vi "Main_MaintenanceCountersV1.vi"() -> ()   [LabVIEW 2017]
panel:
  out "HourResetEnabled":string
  out "CycleCountHour":T1
  in  "ArrayCycleCountHour":T2(array[cluster])
  out "UserLevel":i32
  out "ServerConnectionStatus":string
  out "Line Name":string
  out "Array_BooleanMemoryPLC":T3(array[cluster])
  out "UserLogged":string
  in  "FormatCountersConfigArray":T4(array[cluster]) {"StoppageAlarmCounter" format="%#_6f"; "PreparationAlarmCounter" format="%#_6f"}
  out "CycleTimeCluster":T5
  out "Table Control":string[][](table)
  out "ConnectionCluster":cluster{"Connection":bool, "MachineName":string}
  out "UDT_1":T6
  in  "CountersConfiguration":T7
  out "CountersConfigMerged":T4(array[cluster])
  out "CounterLineName Path":path
  in  "stop":bool
  in  "Tab":T8(tab)
  in  "RefreshLists":bool
  in  "Selector_P#-Description":u16(ring) items=["104567 - Spinning Belt", "108724 - Emergency Stop", "105855 - Helicoil", "101415 - Inductive Sensor", "101111 - Magnetic Sensor"]
  in  "Selector_MachineSpareParts":u16(ring) items=["MA530", "MA520", "MA500-3", "MA500-2", "MA500-1", "MA490-2", "MA490-1", "MA475", "MA470", "MA455", "MA336", "MA335"]
  out "PathLocationMachineImage":path
  out "PathSparePartImage":path
  out "Image_LocationInMachine":T9(plugin-control)
  out "Image_SparePart":T9(plugin-control)
  in  "CountersConfigArray":T4(array[cluster]) {"StoppageAlarmCounter" format="%#_6f"; "PreparationAlarmCounter" format="%#_6f"}
  in  "RefreshCountersConfig":bool
  in  "SaveCountersConfig":bool
  out "Counters Configuration Path":path
  in  "MachineNameID":u16(ring) items=["MA530", "MA520", "MA500-3", "MA500-2", "MA500-1", "MA490-2", "MA490-1", "MA475", "MA470", "MA455", "MA336", "MA335"]
  in  "PLC Connection Array":T10(array[cluster]) {"MemoryType 3" items=["CR (Control Relay)"=1, "MR (Internal Auxiliary Relay)"=2, "VB (Work Relay)"=3, "LR (Latch Relay)"=4, "B (Link Relay)"=5, "R (Relay)"=6, "DM (Data Memory)"=7, "EM (Extended Data Memory)"=8, "FM (File Register 1)"=9, "ZF (FIle Register 2)"=10, "W (Link Register)"=11, "TM (Temporary Data Memory)"=12, "Z (Index Register)"=13, "T (Timer)"=14, "TC (Timer (Counter Value))"=15, "TS (Timer Set Value)"=16, "C (Counter)"=17, "CC (Counter (Counter Value))"=18, "CS (Counter (Set Value))"=19, "CTH (High Speed Counter)"=20, "CTC (High Speed Counter Comparator (Set Value))"=21, "AT (Digital Trimmer)"=22, "CM (Control Memory)"=23, "VM (Work Memory)"=24]; "MemoryType 2" items=["CR (Control Relay)"=1, "MR (Internal Auxiliary Relay)"=2, "VB (Work Relay)"=3, "LR (Latch Relay)"=4, "B (Link Relay)"=5, "R (Relay)"=6, "DM (Data Memory)"=7, "EM (Extended Data Memory)"=8, "FM (File Register 1)"=9, "ZF (FIle Register 2)"=10, "W (Link Register)"=11, "TM (Temporary Data Memory)"=12, "Z (Index Register)"=13, "T (Timer)"=14, "TC (Timer (Counter Value))"=15, "TS (Timer Set Value)"=16, "C (Counter)"=17, "CC (Counter (Counter Value))"=18, "CS (Counter (Set Value))"=19, "CTH (High Speed Counter)"=20, "CTC (High Speed Counter Comparator (Set Value))"=21, "AT (Digital Trimmer)"=22, "CM (Control Memory)"=23, "VM (Work Memory)"=24]; "MemoryType" items=["CR (Control Relay)"=1, "MR (Internal Auxiliary Relay)"=2, "VB (Work Relay)"=3, "LR (Latch Relay)"=4, "B (Link Relay)"=5, "R (Relay)"=6, "DM (Data Memory)"=7, "EM (Extended Data Memory)"=8, "FM (File Register 1)"=9, "ZF (FIle Register 2)"=10, "W (Link Register)"=11, "TM (Temporary Data Memory)"=12, "Z (Index Register)"=13, "T (Timer)"=14, "TC (Timer (Counter Value))"=15, "TS (Timer Set Value)"=16, "C (Counter)"=17, "CC (Counter (Counter Value))"=18, "CS (Counter (Set Value))"=19, "CTH (High Speed Counter)"=20, "CTC (High Speed Counter Comparator (Set Value))"=21, "AT (Digital Trimmer)"=22, "CM (Control Memory)"=23, "VM (Work Memory)"=24]; "PLC Type" items=["Keyence", "Allen Bradley", "Mitsubishi", "Panasonic", "Siemens"]}
  out "PLC Configuration Path":path
  in  "SavePLCConfig":bool
  in  "RefreshPLCConfig":bool
  in  "CreateTables":bool
  in  "EditUser":bool
  in  "GeneralParametersArray":cluster{"Parameter":string, "Value":string}[](array[cluster])
  in  "LoadDefaultConfig":bool
  in  "RemoveUser":bool
  in  "Logout":bool
  in  "Login":bool
  in  "AddUser":bool
  in  "GDrive":bool
  out "GeneralConfigPath":path
  in  "RefreshGeneralConfig":bool
  in  "SaveGeneralConfig":bool
  in  "ShowParetto":bool
  out "CycleTimeMonitor":T11(array[cluster])
  out "CycleTimePath":path
  out "legend":string[][](table)
  in  "Tab Control":T12(tab)
  in  "DictionaryArray":T13(array[cluster]) {"LifeCycle" format="%#_6f"}
  out "PathDictionary":path
  in  "SaveDictionary":bool
  in  "RefreshDictionary":bool
  in  "ResetAlarmButton":bool
  in  "QualityLogin":bool
  in  "MaintenanceLogin":bool
  in  "ResetAlarm":bool[](array[boolean])
  out "ArrayAlarm":bool[](array[boolean])
  out "OnlineStations":T14(array[cluster])
  in  "Counters Monitor Array":T15(array[cluster])
  out "CurrentCountersPath":path
  in  "Count Signal":bool[](array[boolean])
  in  "SaveCurrentCounter":bool
  in  "RefreshCurrentCounter":bool
  in  "Sort":bool
  out "Hour":string
  # "Cycles Based Maintenance"
  # "1. Save counters to be loaded in the last state when the app starts up.\n\n2.Algorithm to read PLC counter values.\nthe key will be to set the signal from the PLC and reset from LabVIEW and the machine won't be able to start the new signal if the application has not been reset the previous one.\n\n3. Autosort getting the red status all the way up.\n\n4. Check cyle time between parts (The count signal must is the same for all the components in the same machine)"
  # "User"
  # "Line"
  # "Nidec Server Connection"
  # "buscar multiplos de ciclos para que coincidan \n\nestudiar investigacion de operaciones\n\nAgrupar las maquinas que trabajan en conjunto para agrupar tareas de mantenimiento.\nCambiar el metodo de seleccion de memorias de PLC usando solo strings para hacerlos universales."
  # "Nota para desarrollador: Revisar que al cerrar la incidencia se apague la alarma y se resetee el contador"
  # "Refresh Lists"
  # "Select Machine"
  # "Select PartNumber - Description"
  # "Spare Part Image"
  # "Location in the Machine"
  # "These paths are calculated automatically"
  # "Machine Name"
  # "Tool Crib P#"
  # "Description"
  # "SP1"
  # "SP2"
  # "Note:\nSP1 = Is the setpoint for the counter when the \nmachine will alert to prepare the replacement of\nthe component. This gives the technician time\nto get parts together.\n\nSP2 = Is the setpoint for the counter when the\nmachine will stop the operation until the part is \nreplaced, the operation can only be reset until\na quality employee comes to unlock with its \nuser and password."
  # "USER LEVEL 3 OR ABOVE TO ENABLE THIS CONFIGURATION IS NEEDED."
  # "Count Signal"
  # "Alarm Signal"
  # "Alarm Message"
  # "Add the option to connect by serial port"
  # "Machine Name"
  # "PLC Address"
  # "PLC Type"
  # "Memory Type"
  # "Number"
  # "Memory Type"
  # "Number"
  # "Number"
  # "Memory Type"
  # "Value"
  # "Parameter"
  # "User Level 5 Requiered to View General Parameters"
  # "User Management"
  # "Idle Time: Is the maximum waiting time before a breakdown incidence is\nconsidered and created."
  # "Escalation Time: Is the maximum waiting time before sending an email \nto the escalation chain."
  # "Cycle Time Monitor"
  # "Cycle Time Monitor"
  # "Note: \nTo add a machine in this list of counters configuration it must be firt added in the PLC Connection tab."
  # "The SubAssembly can be either EOL, Motor, Stator, Rotor Etc, This is used to be able to crate several tables for the same line."
  # "Component"
  # "Cycle Life"
  # "Manual"
  # "Un calculador de tiempo de vida en ciclos, que dependa del tipo de componente para calcular de acuerdo a la aplicacion.\n\npor ejemplo un slider, su tiempo de vida en es km de recorrido, midiendo cuanto se desplaza en cada movimiento, y cuantos desplazamientos hace por ciclo, se puede predecir, a los cuantos\nciclos va a fallar."
  # "Version:\nCBM V1.0\n02/19/2022\nEdgar Cruz\nMaintenance"
  # "Online Stations"
  # "MachineName"
  # "Tool Crib"
  # "ComponentName"
  # "Counter SetPoint"
  # "Actual"
  # "Status"
  # "Maintenance"
  # "Quality"
  # "Current Hour"
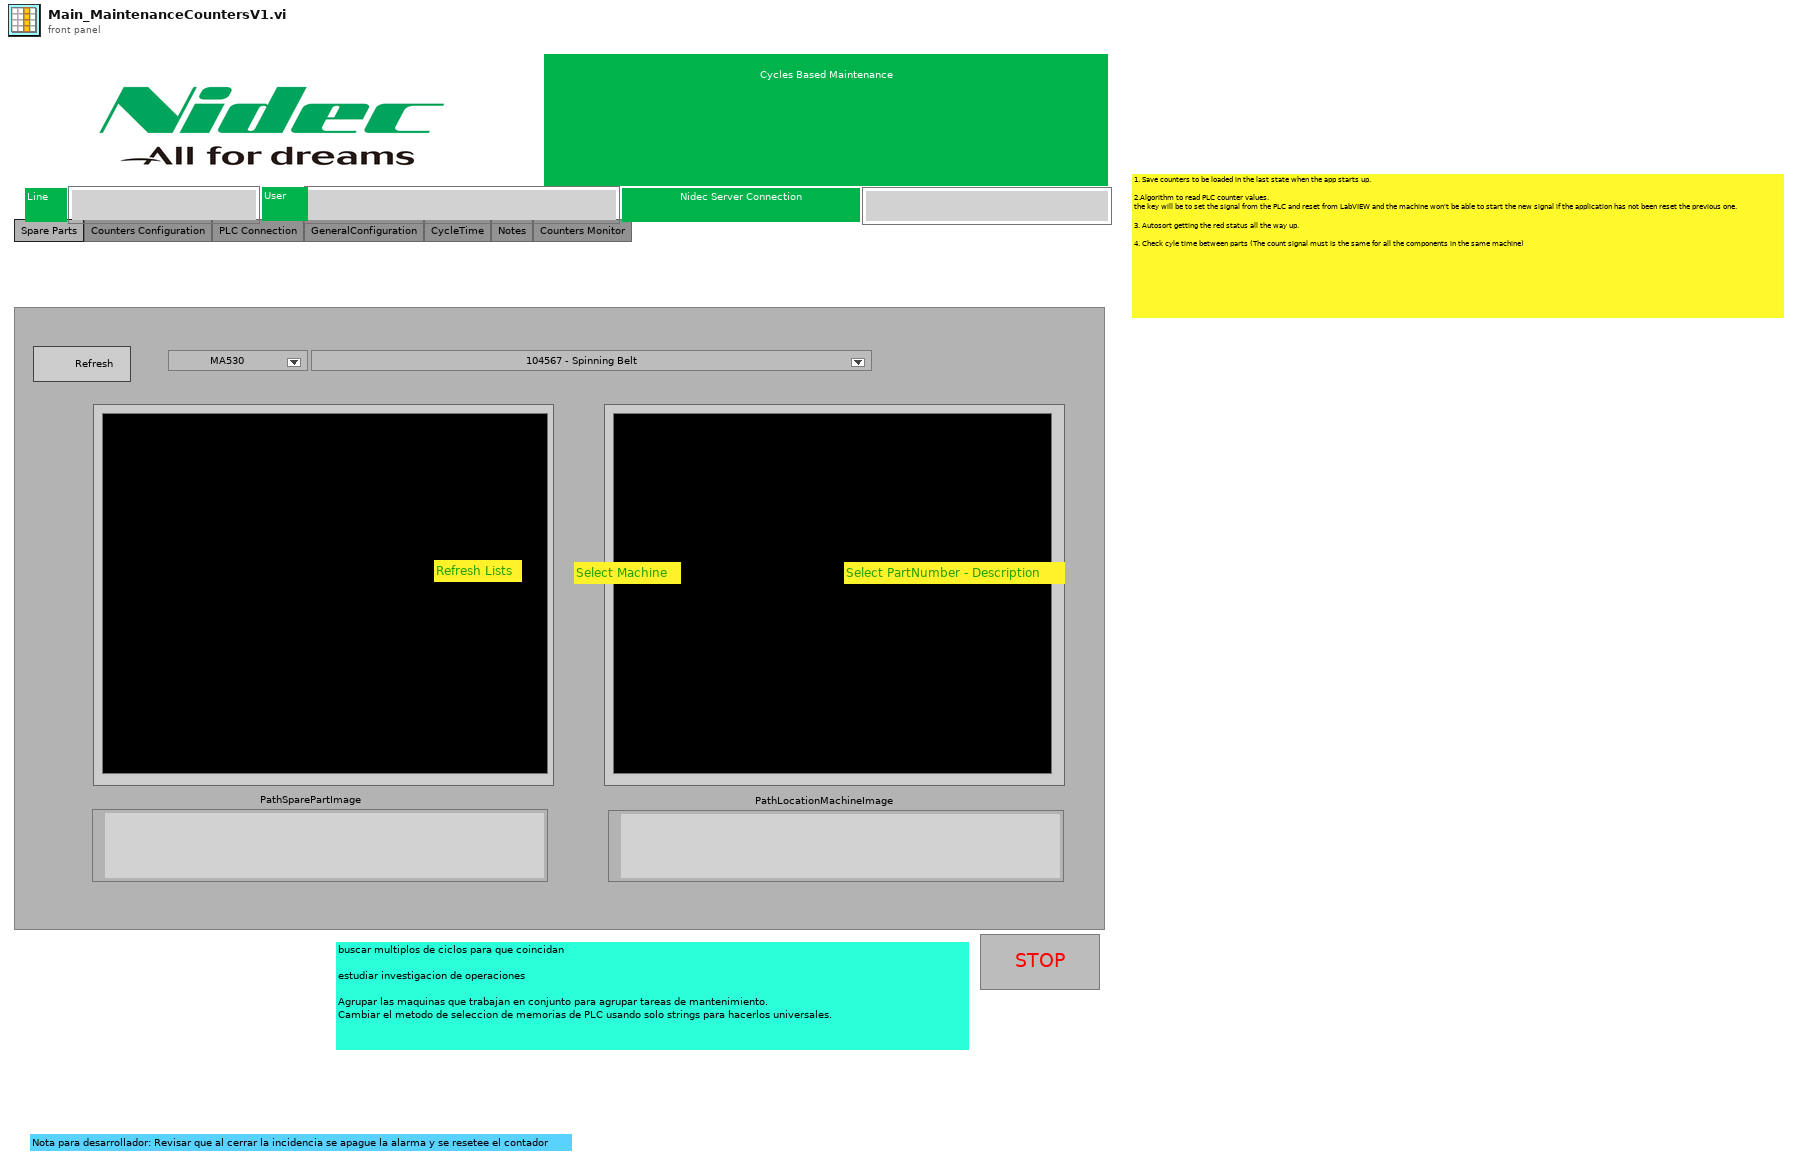
[diagram p1: front panel]
types:
  T1 = cluster{"MachineName":string, "HourLastCycle":string}
  T2 = cluster{"MachineName":string, "HourLastCycle":string}[]
  T3 = cluster{"PLC_Signal":bool, "MachineName":string}[]
  T4 = cluster{"ToolCribPartNumber":string, "ComponentName":string, "PreparationAlarmCounter":dbl, "StoppageAlarmCounter":dbl}[]
  T5 = cluster{"Connection":bool, "MachineName":string, "CycleTime":dbl}
  T6 = cluster{"ToolCribPartNumber":string, "ComponentName":string, "PreparationAlarmCounter":dbl, "StoppageAlarmCounter":dbl, "MachineName":string}
  T7 = cluster{"MachineName":string, "ComponentName":string, "StoppageAlarmCounter":dbl, "CurrentCount":dbl, "StatusColorBox":u32, "ToolCribPartNumber":string}
  T8 = enum32{"Spare Parts", "Counters Configuration", "PLC Connection", "GeneralConfiguration", "CycleTime", "Notes", "Counters Monitor"}
  T9 = typedef "IMAQ Image.ctl" = refnum<image>
  T10 = cluster{"MachineName":string, "PLC Address":string, "PLC Type":u16, "MemoryNumber":i32, "MemoryType":u16, "MemoryType 2":u16, "MemoryNumber 2":i32, "MemoryType 3":u16, "MemoryNumber 3":i32}[]
  T11 = cluster{"Connection":bool, "MachineName":string, "CycleTime":dbl}[]
  T12 = enum32{"Notes", "Dictionary", "Calculator", "Version Information"}
  T13 = cluster{"ComponentDescription":string, "LifeCycle":dbl, "ManualPDF":string}[]
  T14 = cluster{"Connection":bool, "MachineName":string}[]
  T15 = cluster{"MachineName":string, "ComponentName":string, "StoppageAlarmCounter":i32, "CurrentCount":i32, "StatusColorBox":u32, "ToolCribPartNumber":string}[]
  T16 = cluster{"ToolCribPartNumber":string, "ComponentName":string, "PreparationAlarmCounter":dbl, "StoppageAlarmCounter":dbl, "MachineName":string}[]
  T17 = cluster{"MachineName":string, "ComponentName":string, "StoppageAlarmCounter":i32, "CurrentCount":i32, "StatusColorBox":u32, "ToolCribPartNumber":string}
  T18 = enum8{"Enabled", "Disabled", "Disabled and Grayed Out"}
  T19 = typedef "Image Type" = u32
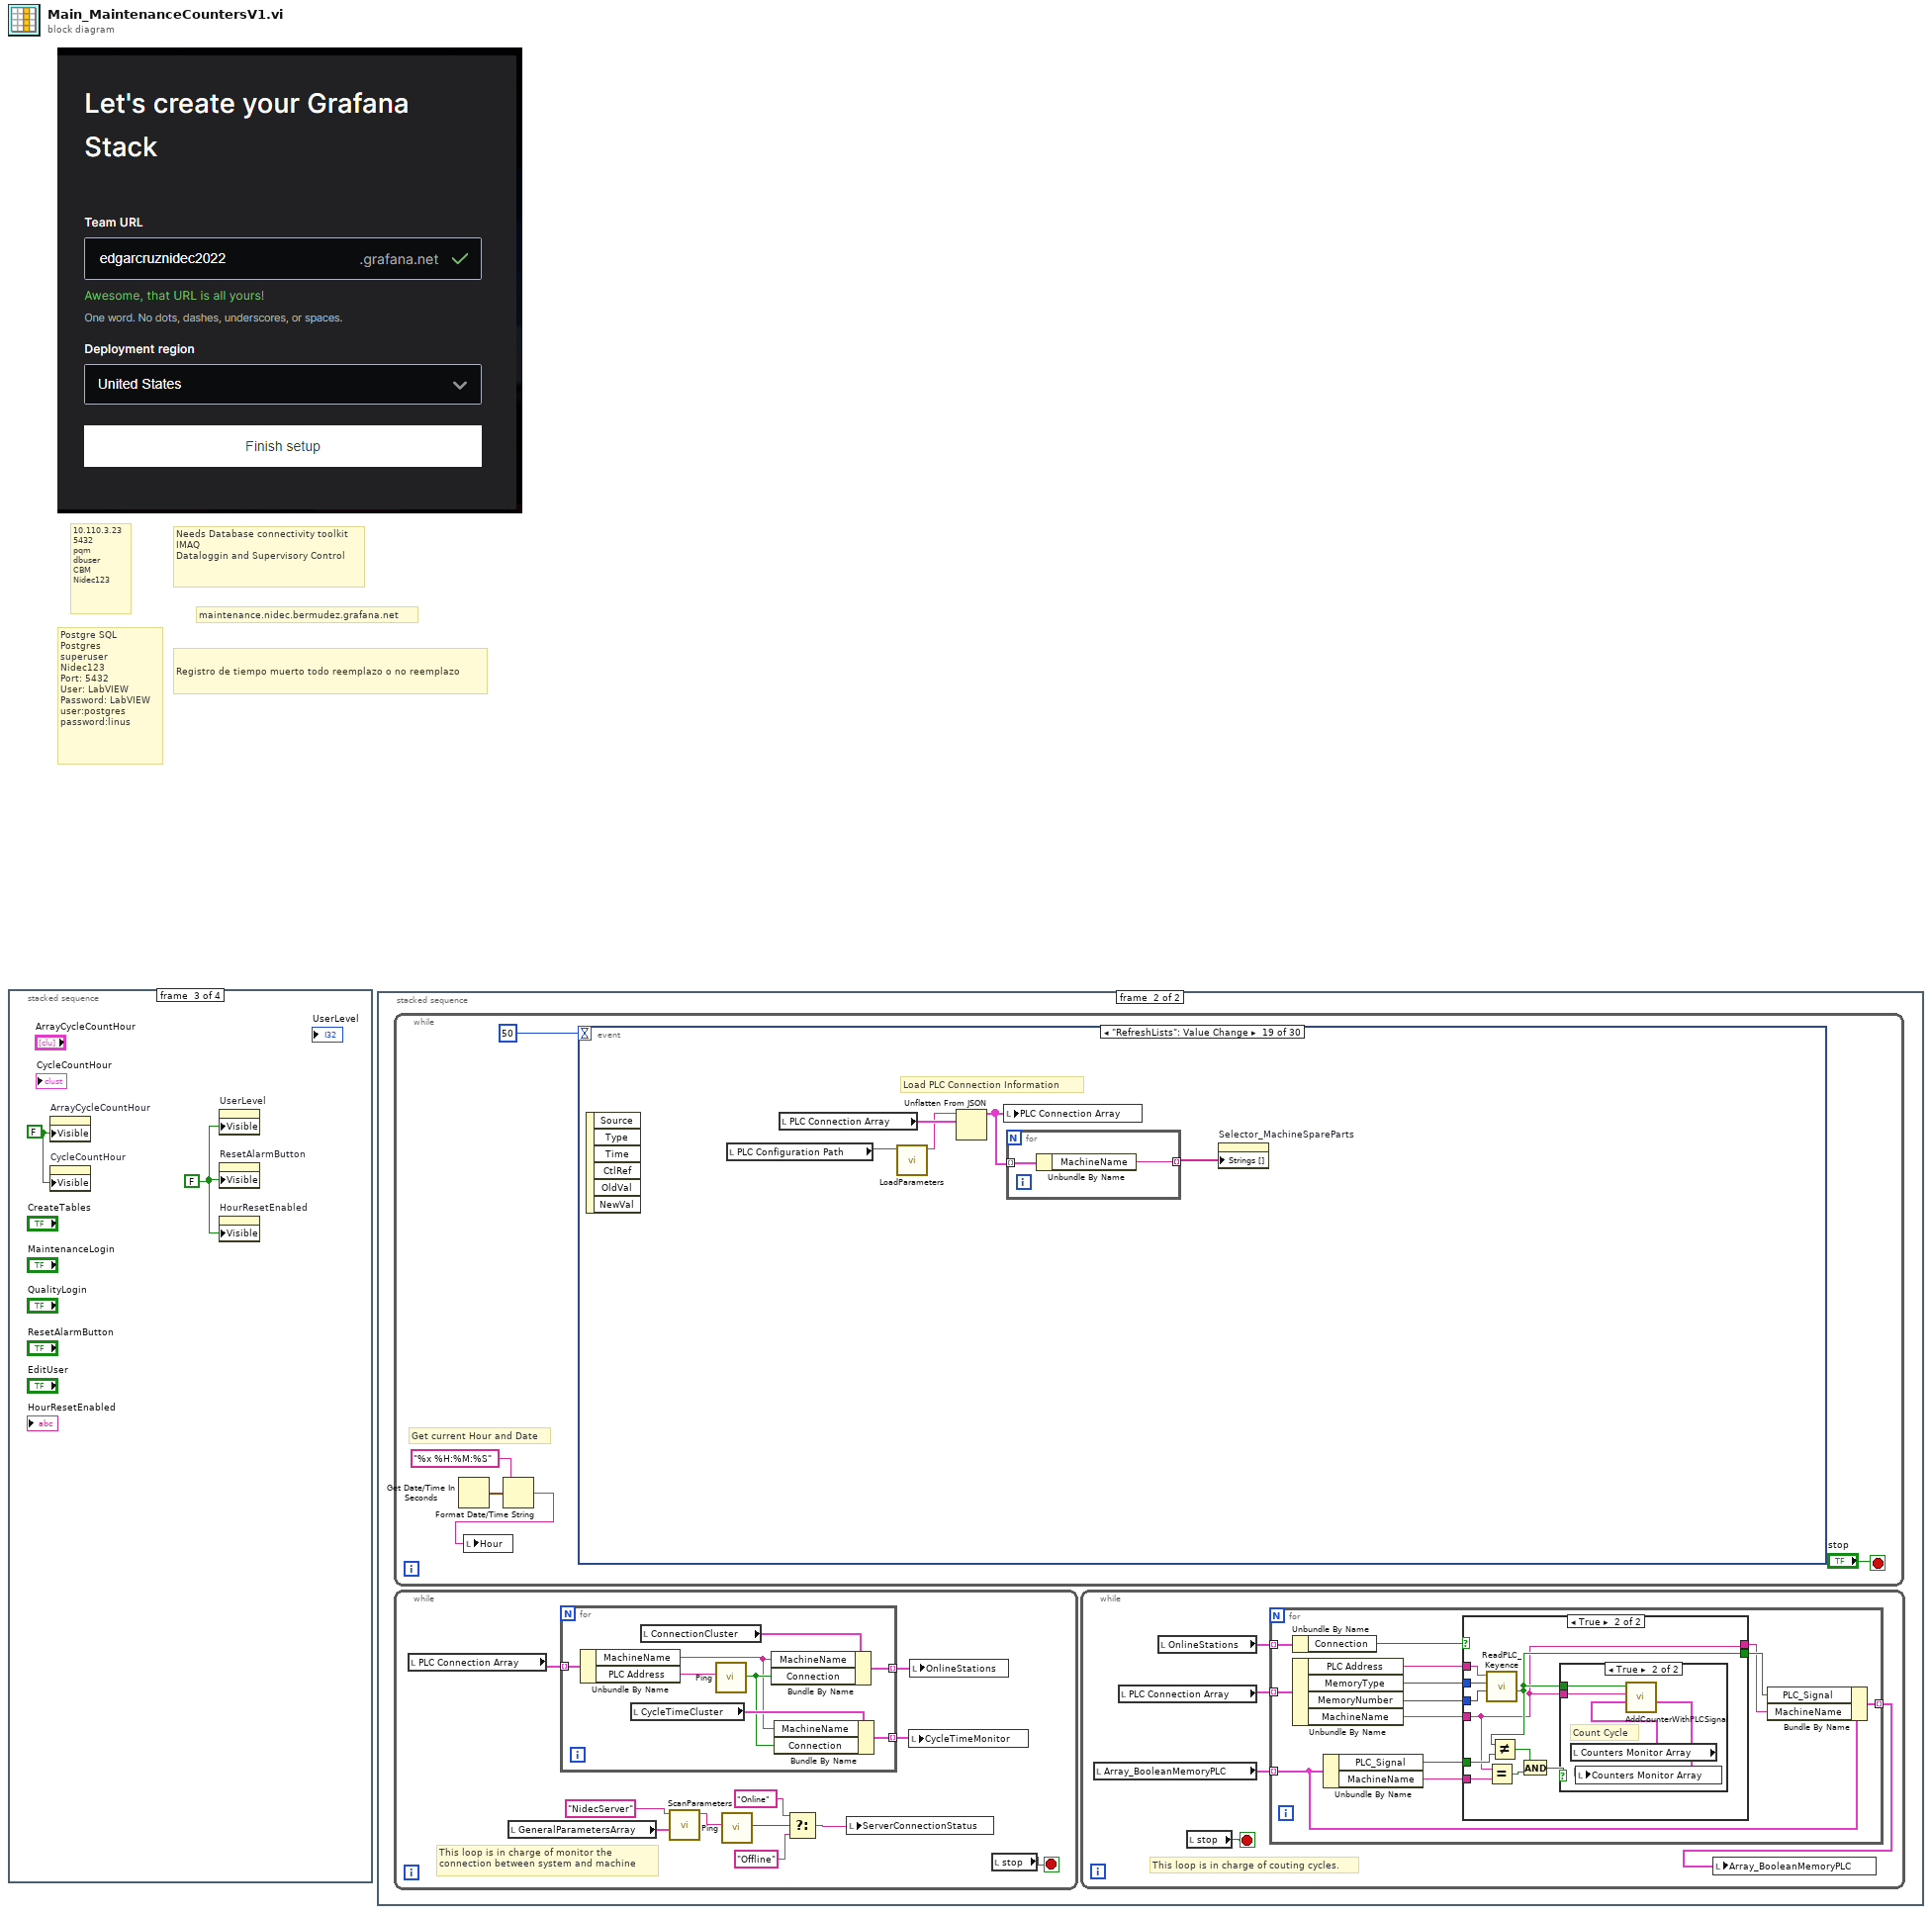
[diagram p0: block diagram]
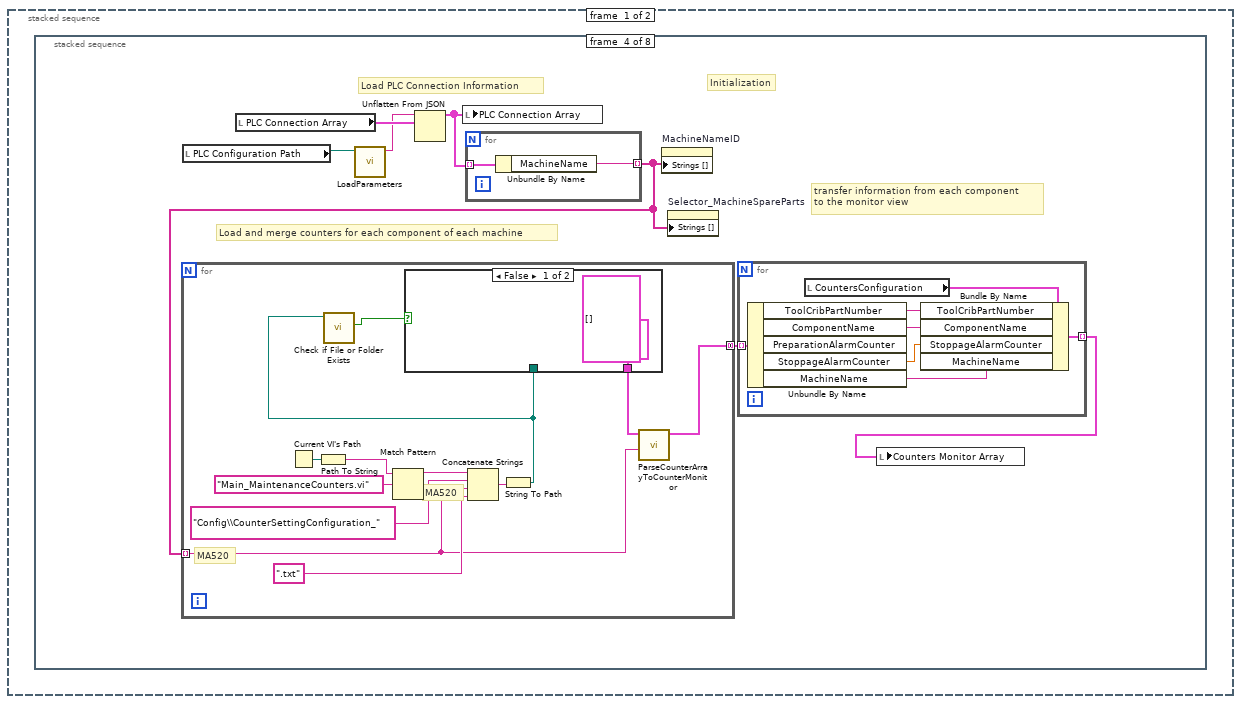
[diagram p2: hidden frame]
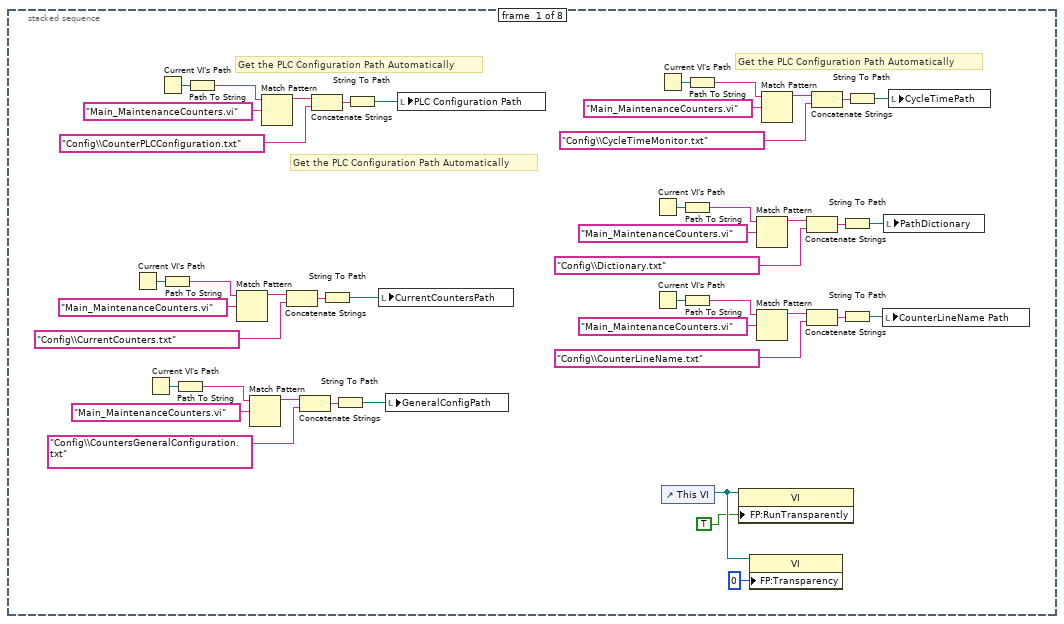
[diagram p3: hidden frame]
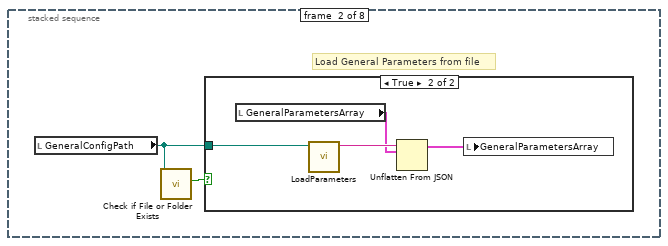
[diagram p4: hidden frame]
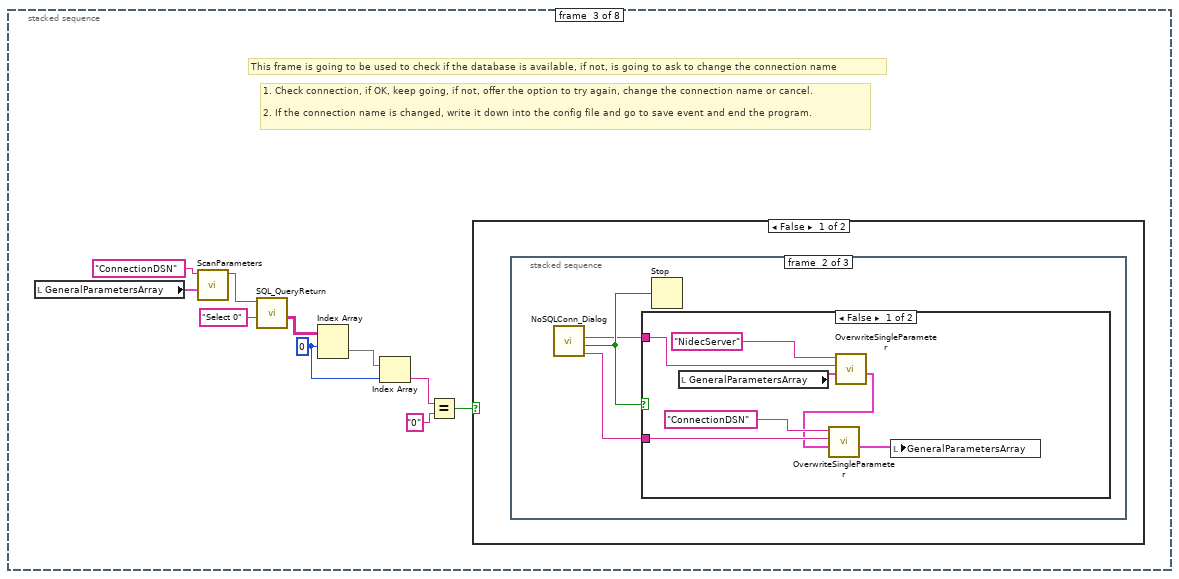
[diagram p6: hidden frame]
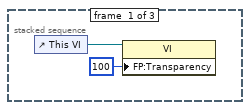
[diagram p7: hidden frame]
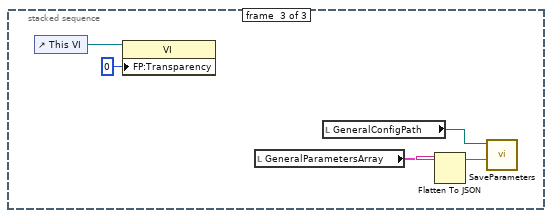
[diagram p9: hidden frame]
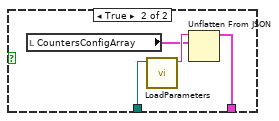
[diagram p11: hidden frame]
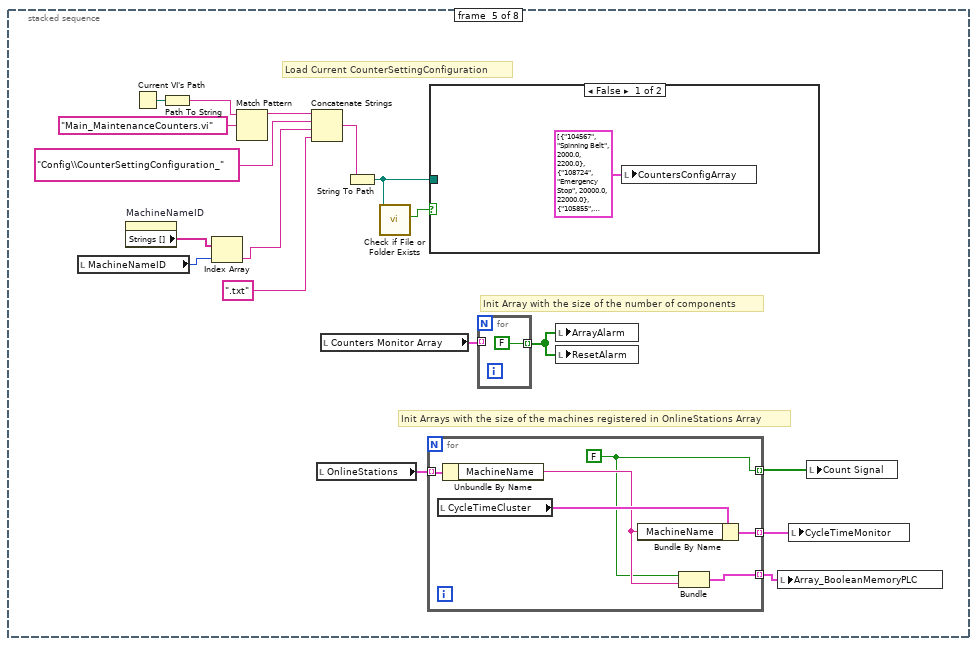
[diagram p12: hidden frame]
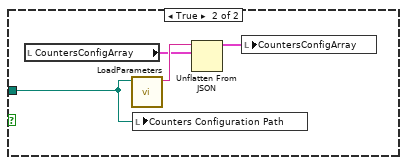
[diagram p13: hidden frame]
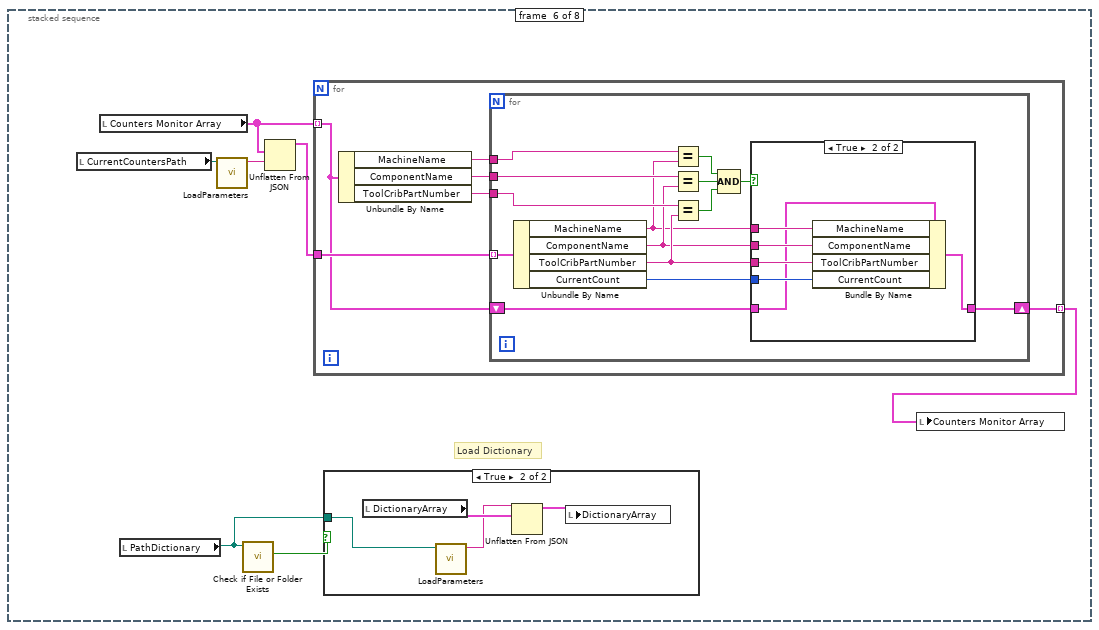
[diagram p14: hidden frame]
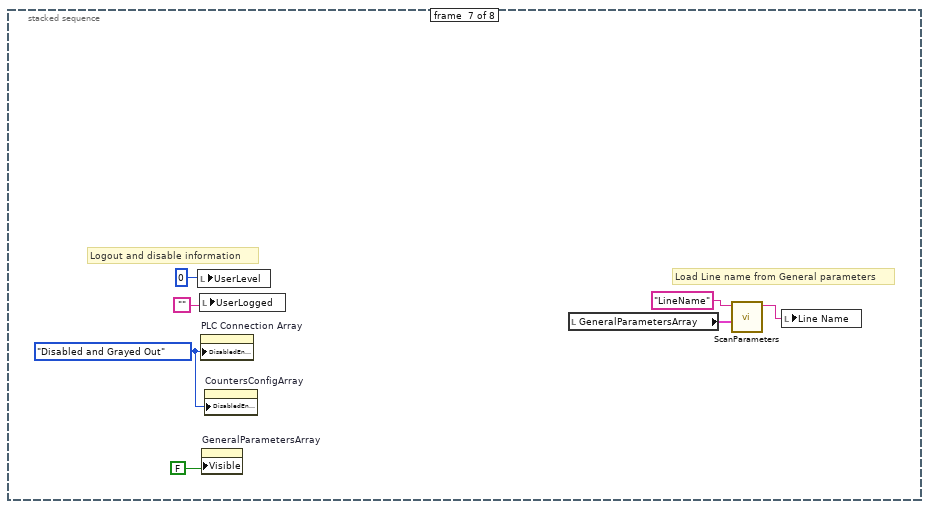
[diagram p17: hidden frame]
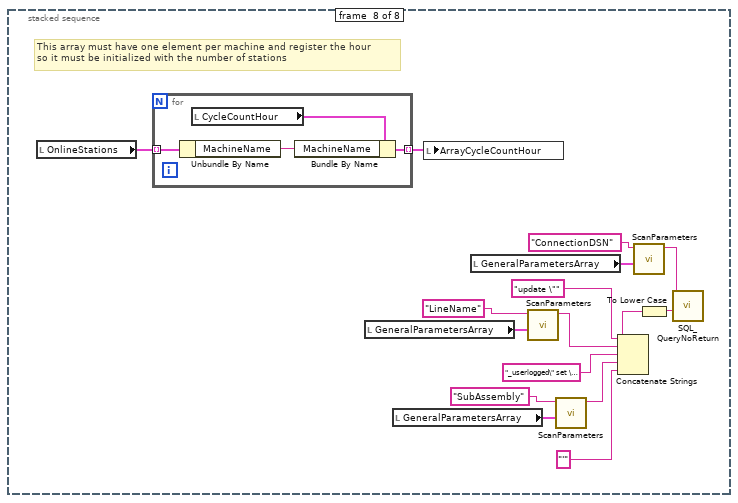
[diagram p18: hidden frame]
diagram:
  # "10.110.3.23\n5432\npqm\ndbuser\nCBM\nNidec123"
  # "maintenance.nidec.bermudez.grafana.net"
  # "Needs Database connectivity toolkit\nIMAQ\nDataloggin and Supervisory Control"
  # "Registro de tiempo muerto todo reemplazo o no reemplazo"
  # "Postgre SQL \nPostgres\nsuperuser\nNidec123\nPort: 5432\nUser: LabVIEW\nPassword: LabVIEW\nuser:postgres\npassword:linus"
  n1 = stacked-sequence {
    frame #0 {
      w5 = FALSE
      # "Main Board"
      n2 = property on="CountersConfiguration" class="Clust (strict)"("Visible"=w5) -> ()  [unwired: 2 in, 2 out]
      n3 = property on="CountersConfigMerged" class="Arr (strict)"("Visible"=w5) -> ()  [unwired: 2 in, 2 out]
      n4 = property on="CounterLineName Path" class="Path"("Visible"=FALSE) -> ()  [unwired: 2 in, 2 out]
      n5 = property on="Count Signal" class="Arr (strict)"("Visible"=FALSE) -> ()  [unwired: 2 in, 2 out]
      n6 = property on="ConnectionCluster" class="Clust (strict)"("Visible"=FALSE) -> ()  [unwired: 2 in, 2 out]
      n7 = local write "stop"(FALSE ("stop")) -> ()
      n8 = property on="UDT_1" class="Clust (strict)"("Visible"=FALSE) -> ()  [unwired: 2 in, 2 out]
    }
    frame #1 {
      w7 = FALSE ("Visible")
      w8 = FALSE ("Visible")
      # "Configuration"
      n9 = property on="CycleTimeCluster" class="Clust (strict)"("Visible"=FALSE) -> ()  [unwired: 2 in, 2 out]
      n10 = property on="FormatCountersConfigArray" class="Arr (strict)"("Visible"=w8) -> ()  [unwired: 2 in, 2 out]
      n11 = property on="Table Control" class="Tbl (strict)"("Visible"=w8) -> ()  [unwired: 2 in, 2 out]
      n12 = property on="Array_BooleanMemoryPLC" class="Arr (strict)"("Visible"=w8) -> ()  [unwired: 2 in, 2 out]
      n13 = property on="ArrayAlarm" class="Arr (strict)"("Visible"=w7) -> ()  [unwired: 2 in, 2 out]
      n14 = property on="ResetAlarm" class="Arr (strict)"("Visible"=w7) -> ()  [unwired: 2 in, 2 out]
      n15 = property on="GDrive" class="Bool"("Visible"=w7) -> ()  [unwired: 2 in, 2 out]
    }
    frame #2 {
      w11 = FALSE
      w10 = FALSE
      n16 = property on="ArrayCycleCountHour" class="Arr (strict)"("Visible"=w11) -> ()  [unwired: 2 in, 2 out]
      n17 = property on="CycleCountHour" class="Clust (strict)"("Visible"=w11) -> ()  [unwired: 2 in, 2 out]
      n18 = property on="UserLevel" class="DigNum (strict)"("Visible"=w10) -> ()  [unwired: 2 in, 2 out]
      n19 = property on="ResetAlarmButton" class="Bool"("Visible"=w10) -> ()  [unwired: 2 in, 2 out]
      n20 = property on="HourResetEnabled" class="Str"("Visible"=w10) -> ()  [unwired: 2 in, 2 out]
    }
    frame #3 {
    }
  }
  n21 = stacked-sequence {
    frame #0 {
      n22 = stacked-sequence {
        frame #0 {
          # "Get the PLC Configuration Path Automatically"
          # "Get the PLC Configuration Path Automatically"
          # "Get the PLC Configuration Path Automatically"
          n23 = Current VI's Path() -> (path=w43:path)
          n24 = Current VI's Path() -> (path=w28:path)
          n25 = Current VI's Path() -> (path=w56:path)
          n26 = Path To String(path=w43) -> (string=w44:string)
          n27 = Path To String(path=w28) -> (string=w27:string)
          n28 = Path To String(path=w56) -> (string=w55:string)
          n29 = Match Pattern(string=w44, regular expression="Main_MaintenanceCounters.vi") -> (before substring=w45:string)  [unwired: 1 in, 3 out]
          n30 = Match Pattern(string=w27, regular expression="Main_MaintenanceCounters.vi") -> (before substring=w26:string)  [unwired: 1 in, 3 out]
          n31 = Match Pattern(string=w55, regular expression="Main_MaintenanceCounters.vi") -> (before substring=w54:string)  [unwired: 1 in, 3 out]
          n32 = Concatenate Strings(w45, "Config\\CurrentCounters.txt" ("regular expression")) -> (w46:string)
          n33 = Concatenate Strings(w26, "Config\\CountersGeneralConfiguration.txt" ("regular expression")) -> (w25:string)
          n34 = Concatenate Strings(w54, "Config\\CounterPLCConfiguration.txt" ("regular expression")) -> (w53:string)
          n35 = String To Path(string=w46) -> (path=w47:path)
          n36 = String To Path(string=w25) -> (path=w22:path)
          n37 = String To Path(string=w53) -> (path=w52:path)
          n38 = local write "CurrentCountersPath"(w47) -> ()
          n39 = local write "GeneralConfigPath"(w22) -> ()
          n40 = local write "PLC Configuration Path"(w52) -> ()
          n41 = Current VI's Path() -> (path=w34:path)
          n42 = Current VI's Path() -> (path=w21:path)
          n43 = Current VI's Path() -> (path=w37:path)
          n44 = control-ref of="This VI"() -> (w14:refnum<vi>)
          n45 = Path To String(path=w34) -> (string=w33:string)
          n46 = Path To String(path=w21) -> (string=w20:string)
          n47 = Path To String(path=w37) -> (string=w38:string)
          n48 = property class="VI"(reference=w14, "FP:RunTransparently"=TRUE) -> ()  [unwired: 1 in, 2 out]
          n49 = property class="VI"(reference=w14, "FP:Transparency"=u8 0 ("Front Panel Window:Transparency")) -> ()  [unwired: 1 in, 2 out]
          n50 = Match Pattern(string=w33, regular expression="Main_MaintenanceCounters.vi") -> (before substring=w32:string)  [unwired: 1 in, 3 out]
          n51 = Match Pattern(string=w20, regular expression="Main_MaintenanceCounters.vi") -> (before substring=w19:string)  [unwired: 1 in, 3 out]
          n52 = Match Pattern(string=w38, regular expression="Main_MaintenanceCounters.vi") -> (before substring=w39:string)  [unwired: 1 in, 3 out]
          n53 = Concatenate Strings(w32, "Config\\Dictionary.txt" ("regular expression")) -> (w31:string)
          n54 = Concatenate Strings(w19, "Config\\CounterLineName.txt" ("regular expression")) -> (w18:string)
          n55 = Concatenate Strings(w39, "Config\\CycleTimeMonitor.txt" ("regular expression")) -> (w40:string)
          n56 = String To Path(string=w31) -> (path=w30:path)
          n57 = String To Path(string=w18) -> (path=w15:path)
          n58 = String To Path(string=w40) -> (path=w41:path)
          n59 = local write "CounterLineName Path"(w15) -> ()
          n60 = local write "PathDictionary"(w30) -> ()
          n61 = local write "CycleTimePath"(w41) -> ()
        }
        frame #1 {
          # "Load General Parameters from file"
          n62 = local read "GeneralConfigPath"() -> (w57:path)
          n63 = call <vilib>:"Check if File or Folder Exists.vi"("path"=w57) -> ("file or folder exists?"=w58:bool)  [unwired: 8 in, 2 out]
          n64 = case shown="True" w58 {
            tunnel: w57 -> [_ w62]
            frame False {
            }
            frame True {
              n65 = local read "GeneralParametersArray"() -> (w60:cluster{"Parameter":string, "Value":string}[])
              n66 = call "LoadParameters.vi"("ShiftConfigPath"=w62) -> ("JSON_Text"=w61:string)  [unwired: 10 in]
              n67 = Unflatten From JSON(JSON string=w61, type and defaults=w60) -> (value=w59:cluster{"Parameter":string, "Value":string}[])  [unwired: 5 in, 1 out]
              n68 = local write "GeneralParametersArray"(w59) -> ()
            }
          }
        }
        frame #2 {
          w65 = 0 ("index (row)")
          # "1. Check connection, if OK, keep going, if not, offer the option to try again, change the connection name or cancel.\n\n2. If the connection name is changed, write it down into the config file and go to save event and end the program."
          # "This frame is going to be used to check if the database is available, if not, is going to ask to change the connection name"
          n69 = local read "GeneralParametersArray"() -> (w72:cluster{"Parameter":string, "Value":string}[])
          n70 = call "ScanParameters.vi"("MainConfigurationArray"=w72, "Parameter"="ConnectionDSN") -> ("Value"=w70:string)  [unwired: 9 in]
          n71 = call "SQL_QueryReturn.vi"("SQL query"="Select 0", "ConnectionDSN"=w70) -> ("data"=w68:string[][])  [unwired: 9 in]
          n72 = Index Array(array=w68, index (row)=w65) -> (element=w66:string[])  [unwired: 1 in]
          n73 = Index Array(array=w66, index=w65) -> (element=w64:string)
          n74 = Equal?(x=w64, y="0" ("SQL query")) -> (x = y?=w63:bool)
          n75 = case shown="False" w63 {
            frame False {
              n76 = stacked-sequence {
                frame #0 {
                  n77 = control-ref of="This VI"() -> (w73:refnum<vi>)
                  n78 = property class="VI"(reference=w73, "FP:Transparency"=u8 100 ("Front Panel Window:Transparency")) -> ()  [unwired: 1 in, 2 out]
                }
                frame #1 {
                  n79 = call "NoSQLConn_Dialog.vi"() -> ("NewDSN"=w77:string, "Boolean"=w76:bool, "NewIPAddress"=w75:string)  [unwired: 9 in]
                  n80 = case shown="False" w76 {
                    tunnel: w77 -> [w83 _]
                    tunnel: w75 -> [w80 _]
                    frame False {
                      n81 = local read "GeneralParametersArray"() -> (w81:cluster{"Parameter":string, "Value":string}[])
                      n82 = call "OverwriteSingleParameter.vi"("MainConfigurationArrayIN"=w81, "Value"=w80, "Parameter"="NidecServer") -> ("MainConfigurationArrayOUT"=w78:cluster{"Parameter":string, "Value":string}[])  [unwired: 8 in]
                      n83 = call "OverwriteSingleParameter.vi"("MainConfigurationArrayIN"=w78, "Value"=w83, "Parameter"="ConnectionDSN") -> ("MainConfigurationArrayOUT"=w79:cluster{"Parameter":string, "Value":string}[])  [unwired: 8 in]
                      n84 = local write "GeneralParametersArray"(w79) -> ()
                    }
                    frame True {
                    }
                  }
                  n85 = Stop(stop? (T)=w76) -> ()
                }
                frame #2 {
                  n86 = control-ref of="This VI"() -> (w89:refnum<vi>)
                  n87 = property class="VI"(reference=w89, "FP:Transparency"=u8 0 ("Front Panel Window:Transparency")) -> ()  [unwired: 1 in, 2 out]
                  n88 = local read "GeneralParametersArray"() -> (w85:cluster{"Parameter":string, "Value":string}[])
                  n89 = local read "GeneralConfigPath"() -> (w87:path)
                  n90 = Flatten To JSON(anything=w85) -> (JSON string=w86:string)  [unwired: 2 in, 1 out]
                  n91 = call "SaveParameters.vi"("JSON_Text"=w86, "ShiftConfigPath"=w87) -> ()  [unwired: 10 in]
                }
              }
            }
            frame True {
            }
          }
        }
        frame #3 {
          # "Initialization"
          # "transfer information from each component\nto the monitor view"
          # "Load and merge counters for each component of each machine"
          # "Load PLC Connection Information"
          n92 = local read "PLC Configuration Path"() -> (w95:path)
          n93 = local read "PLC Connection Array"() -> (w96:T10)
          n94 = call "LoadParameters.vi"("ShiftConfigPath"=w95) -> ("JSON_Text"=w94:string)  [unwired: 10 in]
          n95 = Unflatten From JSON(JSON string=w94, type and defaults=w96) -> (value=w93:T10)  [unwired: 5 in, 1 out]
          n96 = local write "PLC Connection Array"(w93) -> ()
          n97 = for {
            tunnel: w93 -> [w121] mode=indexing
            tunnel: [w122] -> w90 mode=indexing
            n98 = Unbundle By Name(w121) -> ("MachineName"=w122:string)
          }
          n99 = for {
            tunnel: w90 -> [w108] mode=indexing
            tunnel: [w107] -> w91 mode=concatenating
            # "MA520"
            # "MA520"
            n100 = Current VI's Path() -> (path=w112:path)
            n101 = Path To String(path=w112) -> (string=w113:string)
            n102 = Match Pattern(string=w113, regular expression="Main_MaintenanceCounters.vi") -> (before substring=w114:string)  [unwired: 1 in, 3 out]
            n103 = Concatenate Strings(w114, "Config\\CounterSettingConfiguration_" ("regular expression"), w108, ".txt" ("regular expression")) -> (w115:string)
            n104 = String To Path(string=w115) -> (path=w106:path)
            n105 = call <vilib>:"Check if File or Folder Exists.vi"("path"=w106) -> ("file or folder exists?"=w105:bool)  [unwired: 8 in, 2 out]
            n106 = case shown="False" w105 {
              tunnel: [T4 [] ("CountersConfigArray") w119] -> w104
              tunnel: w106 -> [_ w118]
              frame False {
              }
              frame True {
                n107 = local read "CountersConfigArray"() -> (w117:T4)
                n108 = call "LoadParameters.vi"("ShiftConfigPath"=w118) -> ("JSON_Text"=w120:string)  [unwired: 10 in]
                n109 = Unflatten From JSON(JSON string=w120, type and defaults=w117) -> (value=w119:T4)  [unwired: 5 in, 1 out]
              }
            }
            n110 = call "ParseCounterArrayToCounterMonitor.vi"("MachineID"=w108, "CountersConfigArray"=w104) -> ("CounterMonitorArray"=w107:T16)  [unwired: 9 in]
          }
          n111 = property on="MachineNameID" class="Ring (strict)"("Strings []"=w90) -> ()  [unwired: 2 in, 2 out]
          n112 = property on="Selector_MachineSpareParts" class="Ring (strict)"("Strings []"=w90) -> ()  [unwired: 2 in, 2 out]
          n113 = for {
            tunnel: [w101] -> w92 mode=indexing
            tunnel: w91 -> [w100] mode=indexing
            n114 = Unbundle By Name(w100) -> ("ToolCribPartNumber"=w99:string, "ComponentName"=w102:string, "StoppageAlarmCounter"=w98:dbl, "MachineName"=w97:string)  [unwired: 1 out]
            n115 = local read "CountersConfiguration"() -> (w103:T7)
            n116 = Bundle By Name(cluster=w103, "ToolCribPartNumber"=w99, "ComponentName"=w102, "StoppageAlarmCounter"=w98, "MachineName"=w97) -> (w101:T7)
          }
          n117 = local write "Counters Monitor Array"(w92) -> ()
        }
        frame #4 {
          # "Load Current CounterSettingConfiguration"
          # "Init Array with the size of the number of components"
          # "Init Arrays with the size of the machines registered in OnlineStations Array"
          n118 = local read "MachineNameID"() -> (w140:u16)
          n119 = property on="MachineNameID" class="Ring (strict)"() -> ("Strings []"=w139:string[])  [unwired: 2 in, 2 out]
          n120 = Current VI's Path() -> (path=w135:path)
          n121 = Path To String(path=w135) -> (string=w136:string)
          n122 = Index Array(array=w139, index=w140) -> (element=w134:string)
          n123 = Match Pattern(string=w136, regular expression="Main_MaintenanceCounters.vi") -> (before substring=w137:string)  [unwired: 1 in, 3 out]
          n124 = Concatenate Strings(w137, "Config\\CounterSettingConfiguration_" ("regular expression"), w134, ".txt" ("regular expression")) -> (w138:string)
          n125 = local read "OnlineStations"() -> (w126:T14)
          n126 = local read "Counters Monitor Array"() -> (w128:T15)
          n127 = String To Path(string=w138) -> (path=w132:path)
          n128 = call <vilib>:"Check if File or Folder Exists.vi"("path"=w132) -> ("file or folder exists?"=w133:bool)  [unwired: 8 in, 2 out]
          n129 = for {
            tunnel: w126 -> [w145] mode=indexing
            tunnel: [w142] -> w125 mode=indexing
            tunnel: [w144] -> w124 mode=indexing
            tunnel: [w141] -> w123 mode=indexing
            w142 = FALSE
            n130 = local read "CycleTimeCluster"() -> (w146:T5)
            n131 = Unbundle By Name(w145) -> ("MachineName"=w143:string)
            n132 = Bundle By Name(cluster=w146, "MachineName"=w143) -> (w144:T5)
            n133 = Bundle(w142, "MachineName"=w143) -> (w141:cluster{bool, "MachineName":string})  [unwired: 1 in]
          }
          n134 = case shown="False" w133 {
            tunnel: w132 -> [_ w151]
            frame False {
              n135 = local write "CountersConfigArray"(T4 [{"ToolCribPartNumber"="104567", "ComponentName"="Spinning Belt", "PreparationAlarmCounter"=2000.0, "StoppageAlarmCounter"=2200.0}, {"ToolCribPartNumber"="108724", "ComponentName"="Emergency Stop", "PreparationAlarmCounter"=20000.0, "StoppageAlarmCounter"=22000.0}, {"ToolCribPartNumber"="105855", "ComponentName"="Helicoil", "PreparationAlarmCounter"=38000.0, "StoppageAlarmCounter"=40000.0}, {"ToolCribPartNumber"="101415", "ComponentName"="NewPart", "PreparationAlarmCounter"=12000.0, "StoppageAlarmCounter"=12300.0}] ("CountersConfigArray")) -> ()
            }
            frame True {
              n136 = local read "CountersConfigArray"() -> (w150:T4)
              n137 = call "LoadParameters.vi"("ShiftConfigPath"=w151) -> ("JSON_Text"=w152:string)  [unwired: 10 in]
              n138 = local write "Counters Configuration Path"(w151) -> ()
              n139 = Unflatten From JSON(JSON string=w152, type and defaults=w150) -> (value=w149:T4)  [unwired: 5 in, 1 out]
              n140 = local write "CountersConfigArray"(w149) -> ()
            }
          }
          n141 = for {
            tunnel: w128 -> [_] mode=indexing
            tunnel: [FALSE] -> w127 mode=indexing
          }
          n142 = local write "ArrayAlarm"(w127) -> ()
          n143 = local write "ResetAlarm"(w127) -> ()
          n144 = local write "Array_BooleanMemoryPLC"(w123) -> ()
          n145 = local write "CycleTimeMonitor"(w124) -> ()
          n146 = local write "Count Signal"(w125) -> ()
        }
        frame #5 {
          # "Load Dictionary"
          n147 = local read "CurrentCountersPath"() -> (w159:path)
          n148 = local read "Counters Monitor Array"() -> (w157:T15)
          n149 = local read "PathDictionary"() -> (w153:path)
          n150 = call "LoadParameters.vi"("ShiftConfigPath"=w159) -> ("JSON_Text"=w158:string)  [unwired: 10 in]
          n151 = call <vilib>:"Check if File or Folder Exists.vi"("path"=w153) -> ("file or folder exists?"=w154:bool)  [unwired: 8 in, 2 out]
          n152 = Unflatten From JSON(JSON string=w158, type and defaults=w157) -> (value=w156:T15)  [unwired: 5 in, 1 out]
          n153 = for {
            tunnel: w157 -> [w165] mode=indexing
            tunnel: w156 -> [w166]
            tunnel: [w164] -> w155 mode=indexing
            n154 = Unbundle By Name(w165) -> ("MachineName"=w169:string, "ComponentName"=w168:string, "ToolCribPartNumber"=w167:string)
            n155 = for {
              tunnel: w169 -> [w182]
              tunnel: w168 -> [w181]
              tunnel: w167 -> [w180]
              tunnel: w166 -> [w183] mode=indexing
              shift-right: [w170] -> w164
              shift-left: w165 -> [w171]
              n156 = Unbundle By Name(w183) -> ("MachineName"=w172:string, "ComponentName"=w173:string, "ToolCribPartNumber"=w174:string, "CurrentCount"=w176:i32)
              n157 = Equal?(x=w182, y=w172) -> (x = y?=w178:bool)
              n158 = Equal?(x=w181, y=w173) -> (x = y?=w179:bool)
              n159 = Equal?(x=w180, y=w174) -> (x = y?=w177:bool)
              n160 = Compound Arithmetic op=AND(w178, w179, w177) -> (w175:bool)
              n161 = case shown="True" w175 {
                tunnel: w176 -> [_ w190]
                tunnel: w174 -> [_ w189]
                tunnel: w173 -> [_ w188]
                tunnel: w172 -> [_ w187]
                tunnel: w171 -> [w184 w186]
                tunnel: [w184 w185] -> w170
                frame False {
                }
                frame True {
                  n162 = Bundle By Name(cluster=w186, "MachineName"=w187, "ComponentName"=w188, "ToolCribPartNumber"=w189, "CurrentCount"=w190) -> (w185:T17)
                }
              }
            }
          }
          n163 = case shown="True" w154 {
            tunnel: w153 -> [_ w162]
            frame False {
            }
            frame True {
              n164 = local read "DictionaryArray"() -> (w163:T13)
              n165 = call "LoadParameters.vi"("ShiftConfigPath"=w162) -> ("JSON_Text"=w161:string)  [unwired: 10 in]
              n166 = Unflatten From JSON(JSON string=w161, type and defaults=w163) -> (value=w160:T13)  [unwired: 5 in, 1 out]
              n167 = local write "DictionaryArray"(w160) -> ()
            }
          }
          n168 = local write "Counters Monitor Array"(w155) -> ()
        }
        frame #6 {
          w195 = T18."Disabled and Grayed Out" ("Disabled")
          # "Logout and disable information"
          # "Load Line name from General parameters"
          n169 = local write "UserLevel"(0) -> ()
          n170 = local write "UserLogged"("") -> ()
          n171 = property on="PLC Connection Array" class="Arr (strict)"("DisabledEnum"=w195) -> ()  [unwired: 2 in, 2 out]
          n172 = property on="GeneralParametersArray" class="Arr (strict)"("Visible"=FALSE) -> ()  [unwired: 2 in, 2 out]
          n173 = property on="CountersConfigArray" class="Arr (strict)"("DisabledEnum"=w195) -> ()  [unwired: 2 in, 2 out]
          n174 = local read "GeneralParametersArray"() -> (w192:cluster{"Parameter":string, "Value":string}[])
          n175 = call "ScanParameters.vi"("MainConfigurationArray"=w192, "Parameter"="LineName") -> ("Value"=w193:string)  [unwired: 9 in]
          n176 = local write "Line Name"(w193) -> ()
        }
        frame #7 {
          # "This array must have one element per machine and register the hour \nso it must be initialized with the number of stations"
          n177 = local read "OnlineStations"() -> (w213:T14)
          n178 = for {
            tunnel: w213 -> [w217] mode=indexing
            tunnel: [w214] -> w212 mode=indexing
            n179 = Unbundle By Name(w217) -> ("MachineName"=w215:string)
            n180 = local read "CycleCountHour"() -> (w216:T1)
            n181 = Bundle By Name(cluster=w216, "MachineName"=w215) -> (w214:T1)
          }
          n182 = local read "GeneralParametersArray"() -> (w205:cluster{"Parameter":string, "Value":string}[])
          n183 = local read "GeneralParametersArray"() -> (w204:cluster{"Parameter":string, "Value":string}[])
          n184 = local write "ArrayCycleCountHour"(w212) -> ()
          n185 = local read "GeneralParametersArray"() -> (w210:cluster{"Parameter":string, "Value":string}[])
          n186 = call "ScanParameters.vi"("MainConfigurationArray"=w205, "Parameter"="LineName") -> ("Value"=w206:string)  [unwired: 9 in]
          n187 = call "ScanParameters.vi"("MainConfigurationArray"=w204, "Parameter"="SubAssembly") -> ("Value"=w207:string)  [unwired: 9 in]
          n188 = Concatenate Strings("update \"", w206, "_userlogged\" set \"useroperations\"='0',\"userquality\"='0' where \"subassembly\"='", w207, "'") -> (w208:string)
          n189 = call "ScanParameters.vi"("MainConfigurationArray"=w210, "Parameter"="ConnectionDSN") -> ("Value"=w211:string)  [unwired: 9 in]
          n190 = To Lower Case(string=w208) -> (all lower case string=w209:string)
          n191 = call "SQL_QueryNoReturn.vi"("SQL query"=w209, "ConnectionDSN"=w211) -> ()  [unwired: 10 in]
        }
      }
    }
    frame #1 {
      n192 = while {
        stop <- "stop" stop-if-true
        # "Get current Hour and Date"
        n193 = Get Date/Time In Seconds() -> (seconds since 1Jan1904=w274:timestamp)
        n194 = Format Date/Time String(time format string (%c)="%x %H:%M:%S", seconds (now)=w274) -> (date/time string=w271:string)  [unwired: 1 in]
        n195 = local write "Hour"(w271) -> ()
        n196 = event shown="[18] \"RefreshLists\": Value Change" {
          selector: _ -> [_ _ _ _ _ _ _ _ _ _ _ _ _ _ _ _ _ _ _ _ _ _ _ _ _ _ _ _ _ _]
          dyn-events: _ -> [_ _ _ _ _ _ _ _ _ _ _ _ _ _ _ _ _ _ _ _ _ _ _ _ _ _ _ _ _ _]
          timeout: 50 -> [_ _ _ _ _ _ _ _ _ _ _ _ _ _ _ _ _ _ _ _ _ _ _ _ _ _ _ _ _ _]
          event Timeout {
            n197 = event-data() -> ()  [unwired: 1 in, 3 out]
            n198 = stacked-sequence {
              frame #0 {
                # "These should be in a Database since this is the most critical data."
                # "Continuously store the Current Counters Montior in a File"
                # "Change the status indicator in the Counters Monitor and Send an Email in case any indicator is Red"
                n199 = local read "Counters Monitor Array"() -> (w297:T15)
                n200 = local read "GeneralParametersArray"() -> (w288:cluster{"Parameter":string, "Value":string}[])
                n201 = local read "GeneralParametersArray"() -> (w278:cluster{"Parameter":string, "Value":string}[])
                n202 = local read "GeneralParametersArray"() -> (w287:cluster{"Parameter":string, "Value":string}[])
                n203 = local read "GeneralParametersArray"() -> (w284:cluster{"Parameter":string, "Value":string}[])
                n204 = local read "GeneralParametersArray"() -> (w292:cluster{"Parameter":string, "Value":string}[])
                n205 = local read "ArrayAlarm"() -> (w294:bool[])
                n206 = local read "Counters Monitor Array"() -> (w298:T15)
                n207 = call "ScanParameters.vi"("MainConfigurationArray"=w288, "Parameter"="SenderMail") -> ("Value"=w283:string)  [unwired: 9 in]
                n208 = call "ScanParameters.vi"("MainConfigurationArray"=w278, "Parameter"="ConnectionDSN") -> ("Value"=w276:string)  [unwired: 9 in]
                n209 = call "ScanParameters.vi"("MainConfigurationArray"=w287, "Parameter"="Password") -> ("Value"=w282:string)  [unwired: 9 in]
                n210 = call "ScanParameters.vi"("MainConfigurationArray"=w284, "Parameter"="IncidenceRecipients") -> ("Value"=w281:string)  [unwired: 9 in]
                n211 = call "ScanParameters.vi"("MainConfigurationArray"=w292, "Parameter"="EmailsEnabled") -> ("Value"=w290:string)  [unwired: 9 in]
                n212 = local read "CurrentCountersPath"() -> (w300:path)
                n213 = local read "PLC Connection Array"() -> (w280:T10)
                n214 = local read "Line Name"() -> (w295:string)
                n215 = local read "OnlineStations"() -> (w279:T14)
                n216 = Flatten To JSON(anything=w298) -> (JSON string=w299:string)  [unwired: 2 in, 1 out]
                n217 = call "SaveParameters.vi"("JSON_Text"=w299, "ShiftConfigPath"=w300) -> ()  [unwired: 10 in]
                n218 = call "CountersVisualization.vi"("Counters Monitor Array IN"=w297, "SenderMail"=w283, "ConnectionDSN"=w276, "Password"=w282, "Recipients"=w281, "ArrayAlarmIN"=w294, "LineName"=w295, "PLC Connection Array"=w280, "OnlineStations"=w279, "EmailsEnabled"=w290) -> ("Counters Monitor Array OUT"=w296:T15, "ArrayAlarmOUT"=w293:bool[])  [unwired: 8 in]
                n219 = local write "Counters Monitor Array"(w296) -> ()
                n220 = local write "ArrayAlarm"(w293) -> ()
              }
              frame #1 {
                # "If the usser logged in is level 5, enables all the configurations"
                n221 = local read "UserLevel"() -> (w304:i32)
                n222 = Equal?(x=w304, y=5) -> (x = y?=w302:bool)
                n223 = property on="GeneralParametersArray" class="Arr (strict)"("Visible"=w302) -> ()  [unwired: 2 in, 2 out]
                n224 = property on="CreateTables" class="Bool"("Visible"=w302) -> ()  [unwired: 2 in, 2 out]
                n225 = property on="EditUser" class="Bool"("Visible"=w302) -> ()  [unwired: 2 in, 2 out]
                n226 = property on="LoadDefaultConfig" class="Bool"("Visible"=w302) -> ()  [unwired: 2 in, 2 out]
                n227 = property on="ResetAlarmButton" class="Bool"() -> ("Visible"=w301:bool)  [unwired: 2 in, 2 out]
                n228 = case shown="True" w301 {
                  frame False {
                  }
                  frame True {
                    n229 = stacked-sequence {
                      seq-local: [w313 _ _] -> [_ w329 _]
                      seq-local: [w309 _ _] -> [_ w328 _]
                      seq-local: [w306 _ _] -> [_ w327 _]
                      seq-local: [w312 _ _] -> [_ w326 _]
                      frame #0 {
                        n230 = local read "HourResetEnabled"() -> (w317:string)
                        n231 = local read "Hour"() -> (w325:string)
                        n232 = call <vilib>:"Space Constant.vi"() -> ("String"=w324:string)
                        n233 = call <vilib>:"Space Constant.vi"() -> ("String"=w318:string)
                        n234 = Match Pattern(string=w325, regular expression=w324) -> (after substring=w323:string)  [unwired: 1 in, 3 out]
                        n235 = Match Pattern(string=w317, regular expression=w318) -> (after substring=w319:string)  [unwired: 1 in, 3 out]
                        n236 = Match Pattern(string=w323, regular expression=":" ("time format string (%c)")) -> (before substring=w321:string, after substring=w311:string)  [unwired: 1 in, 2 out]
                        n237 = Match Pattern(string=w319, regular expression=":" ("time format string (%c)")) -> (before substring=w307:string, after substring=w305:string)  [unwired: 1 in, 2 out]
                        n238 = Match Pattern(string=w311, regular expression=":" ("time format string (%c)")) -> (before substring=w309:string)  [unwired: 1 in, 3 out]
                        n239 = Decimal String To Number(string=w321) -> (number=w316:i32)  [unwired: 2 in, 1 out]
                        n240 = Decimal String To Number(string=w307) -> (number=w315:i32)  [unwired: 2 in, 1 out]
                        n241 = Match Pattern(string=w305, regular expression=":" ("time format string (%c)")) -> (before substring=w306:string)  [unwired: 1 in, 3 out]
                        n242 = Subtract(x=w316, y=w315) -> (x-y=w312:i32)
                        n243 = Equal?(x=w312, y=0) -> (x = y?=w313:bool)
                      }
                      frame #1 {
                        # "Difference in hours"
                        # "Enabled minute"
                        # "Current minute"
                        n244 = case shown="True" w329 {
                          tunnel: w328 -> [w338 w356]
                          tunnel: w327 -> [w339 w355]
                          tunnel: w326 -> [w345 _]
                          frame False {
                            n245 = Match Pattern(string=w339, regular expression=":" ("time format string (%c)")) -> (before substring=w342:string)  [unwired: 1 in, 3 out]
                            n246 = Match Pattern(string=w338, regular expression=":" ("time format string (%c)")) -> (before substring=w343:string)  [unwired: 1 in, 3 out]
                            n247 = Multiply(x=w345, y=60) -> (x*y=w336:i32)
                            n248 = Decimal String To Number(string=w342) -> (number=w337:i32)  [unwired: 2 in, 1 out]
                            n249 = Decimal String To Number(string=w343) -> (number=w335:i32)  [unwired: 2 in, 1 out]
                            n250 = Subtract(x=w336, y=w337) -> (x-y=w334:i32)
                            n251 = Add(x=w334, y=w335) -> (x+y=w333:i32)
                            n252 = Greater Or Equal?(x=5 ("y"), y=w333) -> (x >= y?=w331:bool)
                            n253 = Not(x=w331) -> (.not. x?=w330:bool)
                            n254 = property on="ResetAlarmButton" class="Bool"("Visible"=w330) -> ()  [unwired: 2 in, 2 out]
                          }
                          frame True {
                            n255 = Match Pattern(string=w356, regular expression=":" ("time format string (%c)")) -> (before substring=w353:string)  [unwired: 1 in, 3 out]
                            n256 = Match Pattern(string=w355, regular expression=":" ("time format string (%c)")) -> (before substring=w352:string)  [unwired: 1 in, 3 out]
                            n257 = Decimal String To Number(string=w353) -> (number=w351:i32)  [unwired: 2 in, 1 out]
                            n258 = Decimal String To Number(string=w352) -> (number=w350:i32)  [unwired: 2 in, 1 out]
                            n259 = Subtract(x=w351, y=w350) -> (x-y=w348:i32)
                            n260 = Greater Or Equal?(x=w348, y=5) -> (x >= y?=w347:bool)
                            n261 = Not(x=w347) -> (.not. x?=w346:bool)
                            n262 = property on="ResetAlarmButton" class="Bool"("Visible"=w346) -> ()  [unwired: 2 in, 2 out]
                          }
                        }
                      }
                      frame #2 {
                        n263 = property on="ResetAlarmButton" class="Bool"() -> ("Visible"=w358:bool)  [unwired: 2 in, 2 out]
                        n264 = case shown="False" w358 {
                          frame False {
                            n265 = local read "GeneralParametersArray"() -> (w366:cluster{"Parameter":string, "Value":string}[])
                            n266 = local read "GeneralParametersArray"() -> (w365:cluster{"Parameter":string, "Value":string}[])
                            n267 = local read "GeneralParametersArray"() -> (w371:cluster{"Parameter":string, "Value":string}[])
                            n268 = call "ScanParameters.vi"("MainConfigurationArray"=w366, "Parameter"="LineName") -> ("Value"=w367:string)  [unwired: 9 in]
                            n269 = call "ScanParameters.vi"("MainConfigurationArray"=w365, "Parameter"="SubAssembly") -> ("Value"=w368:string)  [unwired: 9 in]
                            n270 = Concatenate Strings("update \"", w367, "_userlogged\" set \"useroperations\"='0',\"userquality\"='0' where \"subassembly\"='", w368, "'") -> (w369:string)
                            n271 = call "ScanParameters.vi"("MainConfigurationArray"=w371, "Parameter"="ConnectionDSN") -> ("Value"=w372:string)  [unwired: 9 in]
                            n272 = To Lower Case(string=w369) -> (all lower case string=w370:string)
                            n273 = call "SQL_QueryNoReturn.vi"("SQL query"=w370, "ConnectionDSN"=w372) -> ()  [unwired: 10 in]
                          }
                          frame True {
                          }
                        }
                      }
                    }
                  }
                }
              }
            }
          }
          event "stop": Value Change {
            n274 = event-data() -> ()  [unwired: 1 in, 6 out]
            n275 = Stop() -> ()  [unwired: 1 in]
          }
          event "SavePLCConfig": Value Change {
            # "Store the PLC Configuration in JSON File"
            n276 = event-data() -> ()  [unwired: 1 in, 6 out]
            n277 = local read "PLC Connection Array"() -> (w384:T10)
            n278 = local read "PLC Configuration Path"() -> (w383:path)
            n279 = Flatten To JSON(anything=w384) -> (JSON string=w382:string)  [unwired: 2 in, 1 out]
            n280 = local read "GeneralParametersArray"() -> (w378:cluster{"Parameter":string, "Value":string}[])
            n281 = local read "GeneralParametersArray"() -> (w374:cluster{"Parameter":string, "Value":string}[])
            n282 = call "SaveParameters.vi"("JSON_Text"=w382, "ShiftConfigPath"=w383) -> ()  [unwired: 10 in]
            n283 = call "ScanParameters.vi"("MainConfigurationArray"=w378, "Parameter"="ConnectionDSN") -> ("Value"=w376:string)  [unwired: 9 in]
            n284 = call "ScanParameters.vi"("MainConfigurationArray"=w374, "Parameter"="LineName") -> ("Value"=w373:string)  [unwired: 9 in]
            n285 = for {
              tunnel: w384 -> [w388] mode=indexing
              tunnel: [w385] -> w379 mode=indexing
              tunnel: w376 -> [w387]
              tunnel: w373 -> [w386]
              # "Disabled because the \ntables have not been \ncreated"
              n286 = Unbundle By Name(w388) -> ("MachineName"=w385:string)
              n287 = disable-structure shown="Disabled" {
                disable-tunnel: w387 -> [w392 _]
                disable-tunnel: w386 -> [w390 _]
                disable-tunnel: w385 -> [w389 _]
                frame Disabled {
                  n288 = call "SQL_CycleTime_RegisterMachine.vi"("MachineName"=w389, "LineName"=w390, "TableName"="CycleTime", "ConnectionDSN"=w392) -> ()  [unwired: 8 in]
                }
                frame Enabled {
                }
              }
            }
            n289 = local read "CounterLineName Path"() -> (w380:path)
            n290 = local read "Line Name"() -> (w381:string)
            n291 = call "SaveParameters.vi"("JSON_Text"=w381, "ShiftConfigPath"=w380) -> ()  [unwired: 10 in]
            n292 = property on="MachineNameID" class="Ring (strict)"("Strings []"=w379) -> ()  [unwired: 2 in, 2 out]
            n293 = property on="Selector_MachineSpareParts" class="Ring (strict)"("Strings []"=w379) -> ()  [unwired: 2 in, 2 out]
          }
          event "RefreshCountersConfig": Value Change {
            n294 = event-data() -> ()  [unwired: 1 in, 6 out]
            n295 = local read "MachineNameID"() -> (w404:u16)
            n296 = property on="MachineNameID" class="Ring (strict)"() -> ("Strings []"=w403:string[])  [unwired: 2 in, 2 out]
            n297 = Current VI's Path() -> (path=w399:path)
            n298 = Path To String(path=w399) -> (string=w400:string)
            n299 = Index Array(array=w403, index=w404) -> (element=w398:string)
            n300 = Match Pattern(string=w400, regular expression="Main_MaintenanceCounters.vi") -> (before substring=w401:string)  [unwired: 1 in, 3 out]
            n301 = Concatenate Strings(w401, "Config\\CounterSettingConfiguration_" ("regular expression"), w398, ".txt" ("regular expression")) -> (w402:string)
            n302 = String To Path(string=w402) -> (path=w393:path)
            n303 = call <vilib>:"Check if File or Folder Exists.vi"("path"=w393) -> ("file or folder exists?"=w394:bool)  [unwired: 8 in, 2 out]
            n304 = case shown="True" w394 {
              tunnel: w393 -> [_ w408]
              frame False {
                n305 = local write "CountersConfigArray"(T4 [] ("CountersConfigArray")) -> ()
              }
              frame True {
                n306 = local read "CountersConfigArray"() -> (w407:T4)
                n307 = call "LoadParameters.vi"("ShiftConfigPath"=w408) -> ("JSON_Text"=w409:string)  [unwired: 10 in]
                n308 = local write "Counters Configuration Path"(w408) -> ()
                n309 = Unflatten From JSON(JSON string=w409, type and defaults=w407) -> (value=w406:T4)  [unwired: 5 in, 1 out]
                n310 = local write "CountersConfigArray"(w406) -> ()
              }
            }
          }
          event "LoadDefaultConfig": Value Change {
            n311 = event-data() -> ()  [unwired: 1 in, 6 out]
            n312 = local write "GeneralParametersArray"(cluster{"Parameter":string, "Value":string}[] [{"Parameter"="SenderMail", "Value"="maintenance.nidec.bermudez@gmail.com"}, {"Parameter"="Password", "Value"="Nidec123"}, {"Parameter"="IncidenceRecipients", "Value"="edgar.cruz@nidec.com"}, {"Parameter"="LineName", "Value"="EPSL3"}, {"Parameter"="ConnectionDSN", "Value"="PostgreSQL30"}, {"Parameter"="UsersTable", "Value"="Users"}, {"Parameter"="NidecServer", "Value"="10.110.3.23"}, {"Parameter"="EmailsEnabled", "Value"="Disabled"}] ("GeneralParametersArray")) -> ()
          }
          event "SaveDictionary": Value Change {
            n313 = event-data() -> ()  [unwired: 1 in, 6 out]
            n314 = local read "DictionaryArray"() -> (w413:T13)
            n315 = local read "PathDictionary"() -> (w411:path)
            n316 = Flatten To JSON(anything=w413) -> (JSON string=w412:string)  [unwired: 2 in, 1 out]
            n317 = call "SaveParameters.vi"("JSON_Text"=w412, "ShiftConfigPath"=w411) -> ()  [unwired: 10 in]
          }
          event "RefreshDictionary": Value Change {
            n318 = event-data() -> ()  [unwired: 1 in, 6 out]
            n319 = local read "PathDictionary"() -> (w414:path)
            n320 = call <vilib>:"Check if File or Folder Exists.vi"("path"=w414) -> ("file or folder exists?"=w415:bool)  [unwired: 8 in, 2 out]
            n321 = case shown="True" w415 {
              tunnel: w414 -> [_ w418]
              frame False {
              }
              frame True {
                n322 = local read "DictionaryArray"() -> (w419:T13)
                n323 = call "LoadParameters.vi"("ShiftConfigPath"=w418) -> ("JSON_Text"=w417:string)  [unwired: 10 in]
                n324 = Unflatten From JSON(JSON string=w417, type and defaults=w419) -> (value=w416:T13)  [unwired: 5 in, 1 out]
                n325 = local write "DictionaryArray"(w416) -> ()
              }
            }
          }
          event "MachineNameID": Value Change {
            n326 = event-data() -> ()  [unwired: 1 in, 6 out]
            n327 = local read "MachineNameID"() -> (w431:u16)
            n328 = property on="MachineNameID" class="Ring (strict)"() -> ("Strings []"=w430:string[])  [unwired: 2 in, 2 out]
            n329 = Current VI's Path() -> (path=w426:path)
            n330 = Path To String(path=w426) -> (string=w427:string)
            n331 = Index Array(array=w430, index=w431) -> (element=w425:string)
            n332 = Match Pattern(string=w427, regular expression="Main_MaintenanceCounters.vi") -> (before substring=w428:string)  [unwired: 1 in, 3 out]
            n333 = Concatenate Strings(w428, "Config\\CounterSettingConfiguration_" ("regular expression"), w425, ".txt" ("regular expression")) -> (w429:string)
            n334 = String To Path(string=w429) -> (path=w420:path)
            n335 = call <vilib>:"Check if File or Folder Exists.vi"("path"=w420) -> ("file or folder exists?"=w421:bool)  [unwired: 8 in, 2 out]
            n336 = case shown="True" w421 {
              tunnel: w420 -> [_ w435]
              frame False {
                n337 = local write "CountersConfigArray"(T4 [] ("CountersConfigArray")) -> ()
              }
              frame True {
                n338 = local read "CountersConfigArray"() -> (w433:T4)
                n339 = call "LoadParameters.vi"("ShiftConfigPath"=w435) -> ("JSON_Text"=w436:string)  [unwired: 10 in]
                n340 = local write "Counters Configuration Path"(w435) -> ()
                n341 = Unflatten From JSON(JSON string=w436, type and defaults=w433) -> (value=w434:T4)  [unwired: 5 in, 1 out]
                n342 = local write "CountersConfigArray"(w434) -> ()
              }
            }
          }
          event "RefreshPLCConfig": Value Change {
            # "Load PLC Connection Information"
            n343 = event-data() -> ()  [unwired: 1 in, 6 out]
            n344 = local read "PLC Configuration Path"() -> (w438:path)
            n345 = local read "PLC Connection Array"() -> (w439:T10)
            n346 = call "LoadParameters.vi"("ShiftConfigPath"=w438) -> ("JSON_Text"=w437:string)  [unwired: 10 in]
            n347 = Unflatten From JSON(JSON string=w437, type and defaults=w439) -> (value=w440:T10)  [unwired: 5 in, 1 out]
            n348 = local write "PLC Connection Array"(w440) -> ()
          }
          event "SaveCountersConfig": Value Change {
            n349 = event-data() -> ()  [unwired: 1 in, 6 out]
            n350 = local read "MachineNameID"() -> (w453:u16)
            n351 = property on="MachineNameID" class="Ring (strict)"() -> ("Strings []"=w452:string[])  [unwired: 2 in, 2 out]
            n352 = Current VI's Path() -> (path=w448:path)
            n353 = Path To String(path=w448) -> (string=w449:string)
            n354 = local read "CountersConfigArray"() -> (w441:T4)
            n355 = Index Array(array=w452, index=w453) -> (element=w445:string)
            n356 = Match Pattern(string=w449, regular expression="Main_MaintenanceCounters.vi") -> (before substring=w450:string)  [unwired: 1 in, 3 out]
            n357 = Concatenate Strings(w450, "Config\\CounterSettingConfiguration_" ("regular expression"), w445, ".txt" ("regular expression")) -> (w451:string)
            n358 = Flatten To JSON(anything=w441) -> (JSON string=w443:string)  [unwired: 2 in, 1 out]
            n359 = String To Path(string=w451) -> (path=w442:path)
            n360 = local write "Counters Configuration Path"(w442) -> ()
            n361 = call "SaveParameters.vi"("JSON_Text"=w443, "ShiftConfigPath"=w442) -> ()  [unwired: 10 in]
          }
          event "Count Signal": Value Change {
            n362 = event-data() -> ()  [unwired: 1 in, 6 out]
            n363 = local read "OnlineStations"() -> (w454:T14)
            n364 = local read "Count Signal"() -> (w455:bool[])
            n365 = for {
              tunnel: w455 -> [w457] mode=indexing
              tunnel: w454 -> [w458] mode=indexing
              n366 = Unbundle By Name(w458) -> ("MachineName"=w456:string)
              n367 = case shown="True" w457 {
                tunnel: w456 -> [_ w460]
                frame False {
                }
                frame True {
                  n368 = local read "Counters Monitor Array"() -> (w461:T15)
                  n369 = for {
                    tunnel: w461 -> [w464] mode=indexing
                    tunnel: w460 -> [w467]
                    tunnel: [w462] -> w459 mode=indexing
                    n370 = Unbundle By Name(w464) -> ("MachineName"=w468:string, "CurrentCount"=w465:i32)
                    n371 = Equal?(x=w467, y=w468) -> (x = y?=w466:bool)
                    n372 = case shown="False" w466 {
                      tunnel: w465 -> [w469 w471]
                      tunnel: [w469 w470] -> w463
                      frame False {
                      }
                      frame True {
                        n373 = Increment(x=w471) -> (x+1=w470:i32)
                      }
                    }
                    n374 = Bundle By Name(cluster=w464, "CurrentCount"=w463) -> (w462:T17)
                  }
                  n375 = local write "Counters Monitor Array"(w459) -> ()
                }
              }
            }
          }
          event "ResetAlarm": Value Change {
            n376 = event-data() -> ()  [unwired: 1 in, 6 out]
            n377 = local read "Counters Monitor Array"() -> (w473:T15)
            n378 = local read "ResetAlarm"() -> (w476:bool[])
            n379 = local read "ArrayAlarm"() -> (w475:bool[])
            n380 = for {
              tunnel: w476 -> [w482] mode=indexing
              tunnel: w475 -> [w479] mode=indexing
              tunnel: [w480] -> w474 mode=indexing
              tunnel: w473 -> [w477] mode=indexing
              tunnel: [w478] -> w472 mode=indexing
              n381 = And(x=w482, y=w479) -> (x .and. y?=w481:bool)
              n382 = case shown="True" w481 {
                tunnel: [w484 FALSE] -> w480
                tunnel: w479 -> [w484 _]
                tunnel: w477 -> [w483 _]
                tunnel: [w483 w488] -> w478
                tunnel: w477 -> [_ w486]
                frame False {
                }
                frame True {
                  n383 = local read "OnlineStations"() -> (w485:T14)
                  n384 = Unbundle By Name(w486) -> ("MachineName"=w487:string)
                  n385 = Bundle By Name(cluster=w486, "CurrentCount"=0) -> (w488:T17)
                  n386 = for {
                    tunnel: w487 -> [w496]
                    tunnel: w485 -> [w498] mode=indexing
                    n387 = Unbundle By Name(w498) -> ("MachineName"=w497:string, "Connection"=w495:bool)
                    n388 = Equal?(x=w495, y=TRUE) -> (x = y?=w493:bool)
                    n389 = Equal?(x=w496, y=w497) -> (x = y?=w492:bool)
                    n390 = And(x=w492, y=w493) -> (x .and. y?=w491:bool)
                    n391 = case shown="True" w491 {
                      tunnel: w496 -> [_ w499]
                      frame False {
                      }
                      frame True {
                        w501 = 0
                        # "Reset the alarm in the PLC"
                        n392 = local read "PLC Connection Array"() -> (w503:T10)
                        n393 = for {
                          tunnel: w503 -> [w519] mode=indexing
                          tunnel: w499 -> [w517]
                          shift-right: [w514] -> w506
                          shift-left: "" -> [w513]
                          shift-right: [w511] -> w504
                          shift-left: w501 -> [w512]
                          shift-right: [w508] -> w505
                          shift-left: w501 -> [w507]
                          n394 = Unbundle By Name(w519) -> ("MachineName"=w518:string, "PLC Address"=w515:string, "MemoryType 2"=w510:u16, "MemoryNumber 2"=w509:i32)
                          n395 = Equal?(x=w517, y=w518) -> (x = y?=w516:bool)
                          n396 = case shown="False" w516 {
                            tunnel: w515 -> [_ w525]
                            tunnel: [w522 w525] -> w514
                            tunnel: w513 -> [w522 _]
                            tunnel: w512 -> [w521 _]
                            tunnel: [w521 w524] -> w511
                            tunnel: w510 -> [_ w524]
                            tunnel: w509 -> [_ w523]
                            tunnel: [w520 w523] -> w508
                            tunnel: w507 -> [w520 _]
                            frame False {
                            }
                            frame True {
                            }
                          }
                        }
                        n397 = call "CBM_WriteBool_PLC_Keyence.vi"("Set?"=FALSE, "MemoryNumber"=w505, "MemoryType"=w504, "PLC_IP"=w506) -> ()  [unwired: 7 in, 1 out]
                      }
                    }
                  }
                }
              }
            }
            n398 = local write "Counters Monitor Array"(w472) -> ()
            n399 = local write "ArrayAlarm"(w474) -> ()
          }
          event "ResetAlarmButton": Value Change {
            n400 = event-data() -> ()  [unwired: 1 in, 6 out]
            n401 = local read "GeneralParametersArray"() -> (w528:cluster{"Parameter":string, "Value":string}[])
            n402 = local read "GeneralParametersArray"() -> (w531:cluster{"Parameter":string, "Value":string}[])
            n403 = local read "Counters Monitor Array"() -> (w536:T15)
            n404 = local read "PLC Connection Array"() -> (w535:T10)
            n405 = local read "OnlineStations"() -> (w537:T14)
            n406 = local read "ArrayAlarm"() -> (w532:bool[])
            n407 = call "ScanParameters.vi"("MainConfigurationArray"=w528, "Parameter"="LineName") -> ("Value"=w526:string)  [unwired: 9 in]
            n408 = call "ScanParameters.vi"("MainConfigurationArray"=w531, "Parameter"="ConnectionDSN") -> ("Value"=w529:string)  [unwired: 9 in]
            n409 = call "ResetAlarm.vi"("LineName"=w526, "ConnectionDSN"=w529, "ArrayAlarmIN"=w532, "PLC Connection Array"=w535, "OnlineStations"=w537, "Counters Monitor Array IN"=w536) -> ("ArrayAlarmOUT"=w533:bool[], "Counters Monitor Array OUT"=w534:T15)  [unwired: 4 in]
            n410 = local write "Counters Monitor Array"(w534) -> ()
            n411 = local write "ArrayAlarm"(w533) -> ()
          }
          event "SaveGeneralConfig": Value Change {
            n412 = event-data() -> ()  [unwired: 1 in, 6 out]
            n413 = local read "GeneralParametersArray"() -> (w538:cluster{"Parameter":string, "Value":string}[])
            n414 = local read "GeneralConfigPath"() -> (w540:path)
            n415 = Flatten To JSON(anything=w538) -> (JSON string=w539:string)  [unwired: 2 in, 1 out]
            n416 = call "SaveParameters.vi"("JSON_Text"=w539, "ShiftConfigPath"=w540) -> ()  [unwired: 10 in]
          }
          event "RefreshGeneralConfig": Value Change {
            n417 = event-data() -> ()  [unwired: 1 in, 6 out]
            n418 = stacked-sequence {
              frame #0 {
                n419 = local read "GeneralConfigPath"() -> (w544:path)
                n420 = local read "GeneralParametersArray"() -> (w542:cluster{"Parameter":string, "Value":string}[])
                n421 = call "LoadParameters.vi"("ShiftConfigPath"=w544) -> ("JSON_Text"=w543:string)  [unwired: 10 in]
                n422 = Unflatten From JSON(JSON string=w543, type and defaults=w542) -> (value=w541:cluster{"Parameter":string, "Value":string}[])  [unwired: 5 in, 1 out]
                n423 = local write "GeneralParametersArray"(w541) -> ()
              }
              frame #1 {
                n424 = local read "GeneralParametersArray"() -> (w546:cluster{"Parameter":string, "Value":string}[])
                n425 = call "ScanParameters.vi"("MainConfigurationArray"=w546, "Parameter"="LineName") -> ("Value"=w547:string)  [unwired: 9 in]
                n426 = local write "Line Name"(w547) -> ()
              }
            }
          }
          event "SaveCurrentCounter": Value Change {
            n427 = event-data() -> ()  [unwired: 1 in, 6 out]
            n428 = local read "Counters Monitor Array"() -> (w548:T15)
            n429 = local read "CurrentCountersPath"() -> (w550:path)
            n430 = Flatten To JSON(anything=w548) -> (JSON string=w549:string)  [unwired: 2 in, 1 out]
            n431 = call "SaveParameters.vi"("JSON_Text"=w549, "ShiftConfigPath"=w550) -> ()  [unwired: 10 in]
          }
          event "RefreshCurrentCounter": Value Change {
            n432 = event-data() -> ()  [unwired: 1 in, 6 out]
            n433 = local read "CurrentCountersPath"() -> (w554:path)
            n434 = local read "Counters Monitor Array"() -> (w552:T15)
            n435 = call "LoadParameters.vi"("ShiftConfigPath"=w554) -> ("JSON_Text"=w553:string)  [unwired: 10 in]
            n436 = Unflatten From JSON(JSON string=w553, type and defaults=w552) -> (value=w551:T15)  [unwired: 5 in, 1 out]
            n437 = local write "Counters Monitor Array"(w551) -> ()
          }
          event "Sort": Value Change {
            n438 = event-data() -> ()  [unwired: 1 in, 6 out]
            n439 = local read "Counters Monitor Array"() -> (w564:T15)
            n440 = for {
              tunnel: w564 -> [w574] mode=indexing
              tunnel: [w573] -> w562 mode=indexing
              tunnel: [w572] -> w561 mode=indexing
              tunnel: [w570] -> w560 mode=indexing
              tunnel: [w568] -> w559 mode=indexing
              tunnel: [w566] -> w558 mode=indexing
              tunnel: [w565] -> w557 mode=indexing
              n441 = Unbundle By Name(w574) -> ("MachineName"=w573:string, "ComponentName"=w572:string, "StoppageAlarmCounter"=w571:i32, "CurrentCount"=w569:i32, "StatusColorBox"=w567:u32, "ToolCribPartNumber"=w565:string)
              n442 = Number To Decimal String(number=w567) -> (decimal integer string=w566:string)  [unwired: 1 in]
              n443 = Number To Decimal String(number=w571) -> (decimal integer string=w570:string)  [unwired: 1 in]
              n444 = Number To Decimal String(number=w569) -> (decimal integer string=w568:string)  [unwired: 1 in]
            }
            n445 = property on="Table Control" class="Tbl (strict)"("Column Headers[]"=string[] ["MachineName", "ComponentName", "StoppageCounter", "CurrentCount", "StatusColorBox", "ToolCribPartNumber"]) -> ()  [unwired: 2 in, 2 out]
            n446 = Build Array(w562, w561, w560, w559, w558, w557) -> (w556:string[][])
            n447 = Transpose 2D Array(2D array=w556) -> (transposed array=w555:string[][])
            n448 = local write "Table Control"(w555) -> ()
          }
          event "RefreshLists": Value Change {
            # "Load PLC Connection Information"
            n449 = event-data() -> ()  [unwired: 1 in, 6 out]
            n450 = local read "PLC Configuration Path"() -> (w577:path)
            n451 = local read "PLC Connection Array"() -> (w578:T10)
            n452 = call "LoadParameters.vi"("ShiftConfigPath"=w577) -> ("JSON_Text"=w576:string)  [unwired: 10 in]
            n453 = Unflatten From JSON(JSON string=w576, type and defaults=w578) -> (value=w575:T10)  [unwired: 5 in, 1 out]
            n454 = local write "PLC Connection Array"(w575) -> ()
            n455 = for {
              tunnel: w575 -> [w580] mode=indexing
              tunnel: [w581] -> w579 mode=indexing
              n456 = Unbundle By Name(w580) -> ("MachineName"=w581:string)
            }
            n457 = property on="Selector_MachineSpareParts" class="Ring (strict)"("Strings []"=w579) -> ()  [unwired: 2 in, 2 out]
          }
          event "Selector_MachineSpareParts": Value Change {
            n458 = event-data() -> ()  [unwired: 1 in, 6 out]
            n459 = local read "Selector_MachineSpareParts"() -> (w593:u16)
            n460 = property on="Selector_MachineSpareParts" class="Ring (strict)"() -> ("Strings []"=w582:string[])  [unwired: 2 in, 2 out]
            n461 = Current VI's Path() -> (path=w589:path)
            n462 = Path To String(path=w589) -> (string=w590:string)
            n463 = Index Array(array=w582, index=w593) -> (element=w588:string)
            n464 = Match Pattern(string=w590, regular expression="Main_MaintenanceCounters.vi") -> (before substring=w591:string)  [unwired: 1 in, 3 out]
            n465 = Concatenate Strings(w591, "Config\\CounterSettingConfiguration_" ("regular expression"), w588, ".txt" ("regular expression")) -> (w592:string)
            n466 = String To Path(string=w592) -> (path=w586:path)
            n467 = call <vilib>:"Check if File or Folder Exists.vi"("path"=w586) -> ("file or folder exists?"=w587:bool)  [unwired: 8 in, 2 out]
            n468 = case shown="True" w587 {
              tunnel: w586 -> [_ w598]
              frame False {
                n469 = local write "CountersConfigArray"(T4 [] ("CountersConfigArray")) -> ()
              }
              frame True {
                n470 = local read "CountersConfigArray"() -> (w597:T4)
                n471 = call "LoadParameters.vi"("ShiftConfigPath"=w598) -> ("JSON_Text"=w599:string)  [unwired: 10 in]
                n472 = Unflatten From JSON(JSON string=w599, type and defaults=w597) -> (value=w595:T4)  [unwired: 5 in, 1 out]
                n473 = for {
                  tunnel: [w602] -> w596 mode=indexing
                  tunnel: w595 -> [w600] mode=indexing
                  n474 = Unbundle By Name(w600) -> ("ToolCribPartNumber"=w605:string, "ComponentName"=w603:string)
                  n475 = call <vilib>:"Space Constant.vi"() -> ("String"=w601:string)
                  n476 = Concatenate Strings(w605, w601, "-", w601, w603) -> (w602:string)
                }
                n477 = property on="Selector_P#-Description" class="Ring (strict)"("Strings []"=w596) -> ()  [unwired: 2 in, 2 out]
              }
            }
          }
          event "Selector_P#-Description": Value Change {
            n478 = event-data() -> ()  [unwired: 1 in, 6 out]
            n479 = stacked-sequence {
              frame #0 {
                w607 = "_"
                n480 = local read "Selector_MachineSpareParts"() -> (w626:u16)
                n481 = local read "Selector_P#-Description"() -> (w624:u16)
                n482 = property on="Selector_MachineSpareParts" class="Ring (strict)"() -> ("Strings []"=w625:string[])  [unwired: 2 in, 2 out]
                n483 = property on="Selector_P#-Description" class="Ring (strict)"() -> ("Strings []"=w623:string[])  [unwired: 2 in, 2 out]
                n484 = Current VI's Path() -> (path=w616:path)
                n485 = Path To String(path=w616) -> (string=w617:string)
                n486 = Index Array(array=w625, index=w626) -> (element=w619:string)
                n487 = Index Array(array=w623, index=w624) -> (element=w612:string)
                n488 = call <vilib>:"Space Constant.vi"() -> ("String"=w611:string)
                n489 = Match Pattern(string=w617, regular expression="Main_MaintenanceCounters.vi") -> (before substring=w618:string)  [unwired: 1 in, 3 out]
                n490 = Concatenate Strings(w618, "Photos\\Spare Parts\\" ("regular expression")) -> (w613:string)
                n491 = Search and Replace String(input string=w612, search string=w611, replace string="") -> (result string=w609:string)  [unwired: 5 in, 3 out]
                n492 = Search and Replace String(input string=w609, search string="-", replace string=w607) -> (result string=w606:string)  [unwired: 5 in, 3 out]
                n493 = Concatenate Strings(w613, w619, w607, w606, ".jpg") -> (w621:string)
                n494 = String To Path(string=w621) -> (path=w620:path)
                n495 = local write "PathSparePartImage"(w620) -> ()
              }
              frame #1 {
                w628 = "_"
                n496 = local read "Selector_MachineSpareParts"() -> (w647:u16)
                n497 = local read "Selector_P#-Description"() -> (w645:u16)
                n498 = property on="Selector_MachineSpareParts" class="Ring (strict)"() -> ("Strings []"=w646:string[])  [unwired: 2 in, 2 out]
                n499 = property on="Selector_P#-Description" class="Ring (strict)"() -> ("Strings []"=w644:string[])  [unwired: 2 in, 2 out]
                n500 = Current VI's Path() -> (path=w637:path)
                n501 = Path To String(path=w637) -> (string=w638:string)
                n502 = Index Array(array=w646, index=w647) -> (element=w640:string)
                n503 = Index Array(array=w644, index=w645) -> (element=w633:string)
                n504 = call <vilib>:"Space Constant.vi"() -> ("String"=w632:string)
                n505 = Match Pattern(string=w638, regular expression="Main_MaintenanceCounters.vi") -> (before substring=w639:string)  [unwired: 1 in, 3 out]
                n506 = Concatenate Strings(w639, "Photos\\Machine Location\\" ("regular expression")) -> (w634:string)
                n507 = Search and Replace String(input string=w633, search string=w632, replace string="") -> (result string=w630:string)  [unwired: 5 in, 3 out]
                n508 = Search and Replace String(input string=w630, search string="-", replace string=w628) -> (result string=w627:string)  [unwired: 5 in, 3 out]
                n509 = Concatenate Strings(w634, w640, w628, w627, ".jpg") -> (w642:string)
                n510 = String To Path(string=w642) -> (path=w641:path)
                n511 = local write "PathLocationMachineImage"(w641) -> ()
              }
              frame #2 {
                n512 = local read "PathLocationMachineImage"() -> (w648:path)
                n513 = local read "PathSparePartImage"() -> (w651:path)
                n514 = call <vilib>:"Check if File or Folder Exists.vi"("path"=w648) -> ("file or folder exists?"=w649:bool)  [unwired: 8 in, 2 out]
                n515 = call <vilib>:"Check if File or Folder Exists.vi"("path"=w651) -> ("file or folder exists?"=w650:bool)  [unwired: 8 in, 2 out]
                n516 = case shown="True" w649 {
                  tunnel: w648 -> [w652 w660]
                  frame False {
                    n517 = Path To String(path=w652) -> (string=w657:string)
                    n518 = Concatenate Strings("La imagen " ("string"), w657, " no existe." ("string")) -> (w656:string)
                    n519 = One Button Dialog(message=w656, button name ("OK")="OK" ("string")) -> ()  [unwired: 1 out]
                  }
                  frame True {
                    w658 = T19 4 items=["Grayscale (U8)", "Grayscale (I16)", "Grayscale (SGL)", "Complex (CSG)", "RGB (U32)", "HSL (U32)", "RGB (U64)", "Grayscale (U16)"] ("Image Type")
                    n520 = call "IMAQ Create"("Image Name"="LocationInMachine", "Image Type"=w658) -> ("New Image"=w662:T9)  [unwired: 3 in, 1 out]
                    n521 = call "IMAQ ReadFile"("File Path"=w660, "Load Color Palette? (No)"=TRUE, "Image"=w662) -> ("Image Out"=w661:T9)  [unwired: 4 in, 4 out]
                    n522 = local write "Image_LocationInMachine"(w661) -> ()
                  }
                }
                n523 = case shown="True" w650 {
                  tunnel: w651 -> [w668 w675]
                  frame False {
                    n524 = Path To String(path=w668) -> (string=w667:string)
                    n525 = Concatenate Strings("La imagen " ("string"), w667, " no existe." ("string")) -> (w665:string)
                    n526 = One Button Dialog(message=w665, button name ("OK")="OK" ("string")) -> ()  [unwired: 1 out]
                  }
                  frame True {
                    w670 = T19 4 items=["Grayscale (U8)", "Grayscale (I16)", "Grayscale (SGL)", "Complex (CSG)", "RGB (U32)", "HSL (U32)", "RGB (U64)", "Grayscale (U16)"] ("Image Type")
                    n527 = call "IMAQ Create"("Image Name"="SparePart", "Image Type"=w670) -> ("New Image"=w673:T9)  [unwired: 3 in, 1 out]
                    n528 = call "IMAQ ReadFile"("File Path"=w675, "Load Color Palette? (No)"=TRUE, "Image"=w673) -> ("Image Out"=w674:T9)  [unwired: 4 in, 4 out]
                    n529 = local write "Image_SparePart"(w674) -> ()
                  }
                }
              }
            }
          }
          event "GDrive": Value Change {
            n530 = event-data() -> ()  [unwired: 1 in, 6 out]
          }
          event "AddUser": Value Change {
            n531 = event-data() -> ()  [unwired: 1 in, 6 out]
            n532 = local read "GeneralParametersArray"() -> (w681:cluster{"Parameter":string, "Value":string}[])
            n533 = local read "GeneralParametersArray"() -> (w678:cluster{"Parameter":string, "Value":string}[])
            n534 = call "ScanParameters.vi"("MainConfigurationArray"=w681, "Parameter"="ConnectionDSN") -> ("Value"=w677:string)  [unwired: 9 in]
            n535 = call "ScanParameters.vi"("MainConfigurationArray"=w678, "Parameter"="UsersTable") -> ("Value"=w676:string)  [unwired: 9 in]
            n536 = call "SQL_CreateUser.vi"("UsersTable"=w676, "ConnectionDSN"=w677) -> ()  [unwired: 10 in]
          }
          event "Login": Value Change {
            w682 = T18."Enabled" ("Disabled")
            n537 = event-data() -> ()  [unwired: 1 in, 6 out]
            n538 = local read "GeneralParametersArray"() -> (w690:cluster{"Parameter":string, "Value":string}[])
            n539 = local read "GeneralParametersArray"() -> (w689:cluster{"Parameter":string, "Value":string}[])
            n540 = call "ScanParameters.vi"("MainConfigurationArray"=w690, "Parameter"="ConnectionDSN") -> ("Value"=w686:string)  [unwired: 9 in]
            n541 = call "ScanParameters.vi"("MainConfigurationArray"=w689, "Parameter"="UsersTable") -> ("Value"=w685:string)  [unwired: 9 in]
            n542 = property on="PLC Connection Array" class="Arr (strict)"("DisabledEnum"=w682) -> ()  [unwired: 2 in, 2 out]
            n543 = property on="CountersConfigArray" class="Arr (strict)"("DisabledEnum"=w682) -> ()  [unwired: 2 in, 2 out]
            n544 = call "SQL_Login.vi"("UsersTable"=w685, "ConnectionDSN"=w686) -> ("qLevel"=w683:i32, "User"=w684:string)  [unwired: 8 in]
            n545 = local write "UserLevel"(w683) -> ()
            n546 = local write "UserLogged"(w684) -> ()
          }
          event "MaintenanceLogin": Value Change {
            n547 = event-data() -> ()  [unwired: 1 in, 6 out]
            n548 = stacked-sequence {
              seq-local: [w691 _] -> [_ w739]
              frame #0 {
                w695 = ","
                n549 = local read "GeneralParametersArray"() -> (w702:cluster{"Parameter":string, "Value":string}[])
                n550 = local read "GeneralParametersArray"() -> (w701:cluster{"Parameter":string, "Value":string}[])
                n551 = call "ScanParameters.vi"("MainConfigurationArray"=w702, "Parameter"="ConnectionDSN") -> ("Value"=w691:string)  [unwired: 9 in]
                n552 = call "ScanParameters.vi"("MainConfigurationArray"=w701, "Parameter"="UsersTable") -> ("Value"=w700:string)  [unwired: 9 in]
                n553 = call "SQL_Login_Maintenance.vi"("UsersTable"=w700, "ConnectionDSN"=w691) -> ("User"=w697:string)  [unwired: 8 in, 1 out]
                n554 = Match Pattern(string=w697, regular expression=w695) -> (after substring=w696:string)  [unwired: 1 in, 3 out]
                n555 = Match Pattern(string=w696, regular expression=w695) -> (before substring=w694:string)  [unwired: 1 in, 3 out]
                n556 = Equal?(x=w694, y="Maintenance") -> (x = y?=w692:bool)
                n557 = case shown="True" w692 {
                  tunnel: w691 -> [_ w714]
                  frame False {
                  }
                  frame True {
                    n558 = local read "GeneralParametersArray"() -> (w712:cluster{"Parameter":string, "Value":string}[])
                    n559 = local read "GeneralParametersArray"() -> (w711:cluster{"Parameter":string, "Value":string}[])
                    n560 = call "ScanParameters.vi"("MainConfigurationArray"=w712, "Parameter"="SubAssembly") -> ("Value"=w705:string)  [unwired: 9 in]
                    n561 = call "ScanParameters.vi"("MainConfigurationArray"=w711, "Parameter"="LineName") -> ("Value"=w708:string)  [unwired: 9 in]
                    n562 = Concatenate Strings("update \"", w708, "_userlogged\" set \"useroperations\"='1' where \"subassembly\"='", w705, "'") -> (w704:string)
                    n563 = To Lower Case(string=w704) -> (all lower case string=w703:string)
                    n564 = call "SQL_QueryNoReturn.vi"("SQL query"=w703, "ConnectionDSN"=w714) -> ()  [unwired: 10 in]
                  }
                }
              }
              frame #1 {
                w718 = "1"
                n565 = local read "GeneralParametersArray"() -> (w738:cluster{"Parameter":string, "Value":string}[])
                n566 = local read "GeneralParametersArray"() -> (w733:cluster{"Parameter":string, "Value":string}[])
                n567 = call "ScanParameters.vi"("MainConfigurationArray"=w738, "Parameter"="LineName") -> ("Value"=w735:string)  [unwired: 9 in]
                n568 = call "ScanParameters.vi"("MainConfigurationArray"=w733, "Parameter"="SubAssembly") -> ("Value"=w731:string)  [unwired: 9 in]
                n569 = Concatenate Strings("select * from \"" ("SQL query"), w735, "_userlogged\" where \"subassembly\"='", w731, "'") -> (w729:string)
                n570 = To Lower Case(string=w729) -> (all lower case string=w728:string)
                n571 = call "SQL_QueryReturn.vi"("SQL query"=w728, "ConnectionDSN"=w739) -> ("data"=w722:string[][])  [unwired: 9 in]
                n572 = Index Array(array=w722, index (col)=2 ("disabled index (col)")) -> (element=w721:string[])  [unwired: 1 in]
                n573 = Index Array(array=w722, index (col)=1 ("disabled index (col)")) -> (element=w726:string[])  [unwired: 1 in]
                n574 = Index Array(array=w721, index=0 ("disabled index (col)")) -> (element=w719:string)
                n575 = Index Array(array=w726, index=0 ("disabled index (col)")) -> (element=w720:string)
                n576 = Equal?(x=w720, y=w718) -> (x = y?=w717:bool)
                n577 = Equal?(x=w718, y=w719) -> (x = y?=w716:bool)
                n578 = And(x=w717, y=w716) -> (x .and. y?=w715:bool)
                n579 = case shown="True" w715 {
                  tunnel: w715 -> [_ w741]
                  frame False {
                  }
                  frame True {
                    n580 = property on="ResetAlarmButton" class="Bool"("Visible"=w741) -> ()  [unwired: 2 in, 2 out]
                    n581 = local read "Hour"() -> (w740:string)
                    n582 = local write "HourResetEnabled"(w740) -> ()
                  }
                }
              }
            }
          }
          event "QualityLogin": Value Change {
            n583 = event-data() -> ()  [unwired: 1 in, 6 out]
            n584 = stacked-sequence {
              seq-local: [w742 _] -> [_ w767]
              frame #0 {
                w745 = ","
                n585 = local read "GeneralParametersArray"() -> (w753:cluster{"Parameter":string, "Value":string}[])
                n586 = local read "GeneralParametersArray"() -> (w752:cluster{"Parameter":string, "Value":string}[])
                n587 = call "ScanParameters.vi"("MainConfigurationArray"=w753, "Parameter"="ConnectionDSN") -> ("Value"=w742:string)  [unwired: 9 in]
                n588 = call "ScanParameters.vi"("MainConfigurationArray"=w752, "Parameter"="UsersTable") -> ("Value"=w751:string)  [unwired: 9 in]
                n589 = call "SQL_Login.vi"("UsersTable"=w751, "ConnectionDSN"=w742) -> ("User"=w750:string)  [unwired: 8 in, 1 out]
                n590 = Match Pattern(string=w750, regular expression=w745) -> (after substring=w749:string)  [unwired: 1 in, 3 out]
                n591 = Match Pattern(string=w749, regular expression=w745) -> (before substring=w748:string)  [unwired: 1 in, 3 out]
                n592 = Equal?(x=w748, y="Quality") -> (x = y?=w747:bool)
                n593 = case shown="True" w747 {
                  tunnel: w742 -> [_ w765]
                  frame False {
                  }
                  frame True {
                    n594 = local read "GeneralParametersArray"() -> (w763:cluster{"Parameter":string, "Value":string}[])
                    n595 = local read "GeneralParametersArray"() -> (w762:cluster{"Parameter":string, "Value":string}[])
                    n596 = call "ScanParameters.vi"("MainConfigurationArray"=w763, "Parameter"="SubAssembly") -> ("Value"=w756:string)  [unwired: 9 in]
                    n597 = call "ScanParameters.vi"("MainConfigurationArray"=w762, "Parameter"="LineName") -> ("Value"=w759:string)  [unwired: 9 in]
                    n598 = Concatenate Strings("update \"", w759, "_userlogged\" set \"userquality\"='1' where \"subassembly\"='", w756, "'") -> (w755:string)
                    n599 = To Lower Case(string=w755) -> (all lower case string=w754:string)
                    n600 = call "SQL_QueryNoReturn.vi"("SQL query"=w754, "ConnectionDSN"=w765) -> ()  [unwired: 10 in]
                  }
                }
              }
              frame #1 {
                w777 = "1"
                n601 = local read "GeneralParametersArray"() -> (w790:cluster{"Parameter":string, "Value":string}[])
                n602 = local read "GeneralParametersArray"() -> (w788:cluster{"Parameter":string, "Value":string}[])
                n603 = call "ScanParameters.vi"("MainConfigurationArray"=w790, "Parameter"="LineName") -> ("Value"=w789:string)  [unwired: 9 in]
                n604 = call "ScanParameters.vi"("MainConfigurationArray"=w788, "Parameter"="SubAssembly") -> ("Value"=w787:string)  [unwired: 9 in]
                n605 = Concatenate Strings("select * from \"" ("SQL query"), w789, "_userlogged\" where \"subassembly\"='", w787, "'") -> (w786:string)
                n606 = To Lower Case(string=w786) -> (all lower case string=w785:string)
                n607 = call "SQL_QueryReturn.vi"("SQL query"=w785, "ConnectionDSN"=w767) -> ("data"=w783:string[][])  [unwired: 9 in]
                n608 = Index Array(array=w783, index (col)=2 ("disabled index (col)")) -> (element=w782:string[])  [unwired: 1 in]
                n609 = Index Array(array=w783, index (col)=1 ("disabled index (col)")) -> (element=w784:string[])  [unwired: 1 in]
                n610 = Index Array(array=w782, index=0 ("disabled index (col)")) -> (element=w780:string)
                n611 = Index Array(array=w784, index=0 ("disabled index (col)")) -> (element=w781:string)
                n612 = Equal?(x=w781, y=w777) -> (x = y?=w779:bool)
                n613 = Equal?(x=w777, y=w780) -> (x = y?=w778:bool)
                n614 = And(x=w779, y=w778) -> (x .and. y?=w766:bool)
                n615 = case shown="True" w766 {
                  selector: w766 -> [_ w791]
                  frame False {
                  }
                  frame True {
                    n616 = local read "Hour"() -> (w792:string)
                    n617 = property on="ResetAlarmButton" class="Bool"("Visible"=w791) -> ()  [unwired: 2 in, 2 out]
                    n618 = local write "HourResetEnabled"(w792) -> ()
                  }
                }
              }
            }
          }
          event "EditUser": Value Change {
            n619 = event-data() -> ()  [unwired: 1 in, 6 out]
            n620 = local read "GeneralParametersArray"() -> (w798:cluster{"Parameter":string, "Value":string}[])
            n621 = local read "GeneralParametersArray"() -> (w797:cluster{"Parameter":string, "Value":string}[])
            n622 = call "ScanParameters.vi"("MainConfigurationArray"=w798, "Parameter"="ConnectionDSN") -> ("Value"=w793:string)  [unwired: 9 in]
            n623 = call "ScanParameters.vi"("MainConfigurationArray"=w797, "Parameter"="UsersTable") -> ("Value"=w794:string)  [unwired: 9 in]
            n624 = call "SQL_EditUser.vi"("UsersTable"=w794, "ConnectionDSN"=w793) -> ()  [unwired: 8 in, 2 out]
          }
          event "Logout": Value Change {
            w814 = T18."Disabled and Grayed Out" ("Disabled")
            n625 = event-data() -> ()  [unwired: 1 in, 6 out]
            n626 = local write "UserLevel"(0) -> ()
            n627 = local write "UserLogged"("") -> ()
            n628 = property on="PLC Connection Array" class="Arr (strict)"("DisabledEnum"=w814) -> ()  [unwired: 2 in, 2 out]
            n629 = property on="ResetAlarmButton" class="Bool"("Visible"=FALSE) -> ()  [unwired: 2 in, 2 out]
            n630 = property on="CountersConfigArray" class="Arr (strict)"("DisabledEnum"=w814) -> ()  [unwired: 2 in, 2 out]
            n631 = local read "GeneralParametersArray"() -> (w806:cluster{"Parameter":string, "Value":string}[])
            n632 = local read "GeneralParametersArray"() -> (w805:cluster{"Parameter":string, "Value":string}[])
            n633 = local read "GeneralParametersArray"() -> (w811:cluster{"Parameter":string, "Value":string}[])
            n634 = call "ScanParameters.vi"("MainConfigurationArray"=w806, "Parameter"="LineName") -> ("Value"=w807:string)  [unwired: 9 in]
            n635 = call "ScanParameters.vi"("MainConfigurationArray"=w805, "Parameter"="SubAssembly") -> ("Value"=w808:string)  [unwired: 9 in]
            n636 = call "ScanParameters.vi"("MainConfigurationArray"=w811, "Parameter"="ConnectionDSN") -> ("Value"=w812:string)  [unwired: 9 in]
            n637 = Concatenate Strings("update \"", w807, "_userlogged\" set \"useroperations\"='0',\"userquality\"='0' where \"subassembly\"='", w808, "'") -> (w809:string)
            n638 = To Lower Case(string=w809) -> (all lower case string=w810:string)
            n639 = call "SQL_QueryNoReturn.vi"("SQL query"=w810, "ConnectionDSN"=w812) -> ()  [unwired: 10 in]
          }
          event "ShowParetto": Value Change {
            n640 = event-data() -> ()  [unwired: 1 in, 6 out]
          }
          event "CreateTables": Value Change {
            n641 = event-data() -> ()  [unwired: 1 in, 6 out]
            n642 = local read "GeneralParametersArray"() -> (w821:cluster{"Parameter":string, "Value":string}[])
            n643 = local read "GeneralParametersArray"() -> (w825:cluster{"Parameter":string, "Value":string}[])
            n644 = local read "GeneralParametersArray"() -> (w819:cluster{"Parameter":string, "Value":string}[])
            n645 = call "ScanParameters.vi"("MainConfigurationArray"=w821, "Parameter"="LineName") -> ("Value"=w820:string)  [unwired: 9 in]
            n646 = call "ScanParameters.vi"("MainConfigurationArray"=w825, "Parameter"="ConnectionDSN") -> ("Value"=w823:string)  [unwired: 9 in]
            n647 = call "ScanParameters.vi"("MainConfigurationArray"=w819, "Parameter"="SubAssembly") -> ("Value"=w817:string)  [unwired: 9 in]
            n648 = call "SQL_CreateTables.vi"("SubAssembly"=w817, "LineName"=w820, "ConnectionDSN"=w823) -> ()  [unwired: 9 in]
          }
        }
      }
      n649 = while {
        stop <- w262 stop-if-true
        # "This loop is in charge of monitor the \nconnection between system and machine"
        n650 = local read "PLC Connection Array"() -> (w260:T10)
        n651 = local read "GeneralParametersArray"() -> (w257:cluster{"Parameter":string, "Value":string}[])
        n652 = for {
          tunnel: w260 -> [w270] mode=indexing
          tunnel: [w267] -> w261 mode=indexing
          tunnel: [w263] -> w259 mode=indexing
          n653 = Unbundle By Name(w270) -> ("MachineName"=w264:string, "PLC Address"=w269:string)
          n654 = local read "CycleTimeCluster"() -> (w266:T5)
          n655 = local read "ConnectionCluster"() -> (w268:cluster{"Connection":bool, "MachineName":string})
          n656 = call "Ping.vi"("hostNameOrAddress"=w269) -> ("bolStatus"=w265:bool)  [unwired: 8 in, 2 out]
          n657 = Bundle By Name(cluster=w268, "MachineName"=w264, "Connection"=w265) -> (w267:cluster{"Connection":bool, "MachineName":string})
          n658 = Bundle By Name(cluster=w266, "MachineName"=w264, "Connection"=w265) -> (w263:T5)
        }
        n659 = call "ScanParameters.vi"("MainConfigurationArray"=w257, "Parameter"="NidecServer") -> ("Value"=w256:string)  [unwired: 9 in]
        n660 = call "Ping.vi"("hostNameOrAddress"=w256) -> ("bolStatus"=w255:bool)  [unwired: 8 in, 2 out]
        n661 = Select(t="Online", s=w255, f="Offline") -> (s? t:f=w254:string)
        n662 = local write "ServerConnectionStatus"(w254) -> ()
        n663 = local write "CycleTimeMonitor"(w259) -> ()
        n664 = local write "OnlineStations"(w261) -> ()
        n665 = local read "stop"() -> (w262:bool)
      }
      n666 = while {
        stop <- w222 stop-if-true
        # "This loop is in charge of couting cycles."
        n667 = local read "Array_BooleanMemoryPLC"() -> (w219:T3)
        n668 = local read "PLC Connection Array"() -> (w220:T10)
        n669 = local read "OnlineStations"() -> (w221:T14)
        n670 = local read "stop"() -> (w222:bool)
        n671 = for {
          tunnel: w221 -> [w235] mode=indexing
          tunnel: w220 -> [w233] mode=indexing
          tunnel: w219 -> [w226] mode=indexing
          tunnel: [w223] -> w218 mode=indexing
          n672 = Unbundle By Name(w235) -> ("Connection"=w234:bool)
          n673 = Unbundle By Name(w233) -> ("PLC Address"=w230:string, "MemoryType"=w231:u16, "MemoryNumber"=w232:i32, "MachineName"=w229:string)
          n674 = Unbundle By Name(w226) -> ("PLC_Signal"=w225:bool, "MachineName"=w224:string)
          n675 = case shown="True" w234 {
            tunnel: w232 -> [_ w247]
            tunnel: w231 -> [_ w246]
            tunnel: w230 -> [_ w245]
            tunnel: w229 -> [_ w241]
            tunnel: [w237 w243] -> w228
            tunnel: [w236 w241] -> w227
            tunnel: w225 -> [w237 w244]
            tunnel: w224 -> [w236 w242]
            frame False {
            }
            frame True {
              n676 = call "ReadPLC_Keyence.vi"("MemoryNumber"=w247, "MemoryType"=w246, "IP Address"=w245) -> ("BoolRead"=w243:bool)  [unwired: 8 in]
              n677 = Equal?(x=w241, y=w242) -> (x = y?=w240:bool)
              n678 = Not Equal?(x=w243, y=w244) -> (x != y?=w239:bool)
              n679 = And(x=w239, y=w240) -> (x .and. y?=w238:bool)
              n680 = case shown="True" w238 {
                tunnel: w243 -> [_ w249]
                tunnel: w241 -> [_ w248]
                frame False {
                }
                frame True {
                  # "Count Cycle"
                  n681 = local read "Counters Monitor Array"() -> (w251:T15)
                  n682 = call "AddCounterWithPLCSignal.vi"("Counters Monitor Array IN"=w251, "MachineName"=w248, "PLC_Bool_IN"=w249) -> ("Counters Monitor Array OUT"=w250:T15)  [unwired: 8 in]
                  n683 = local write "Counters Monitor Array"(w250) -> ()
                }
              }
            }
          }
          n684 = Bundle By Name(cluster=w226, "PLC_Signal"=w228, "MachineName"=w227) -> (w223:cluster{"PLC_Signal":bool, "MachineName":string})
        }
        n685 = local write "Array_BooleanMemoryPLC"(w218) -> ()
      }
    }
  }
